vi "MC_7_12e_JW.vi"() -> ()   [LabVIEW 2011]
uses:
  <vilib>/Utility/file.llb/Read From Spreadsheet File (string).vi
  <vilib>/Utility/inputDevices.llb/keyboardAcquire.vi
  <vilib>/Utility/file.llb/Write To Spreadsheet File (DBL).vi
  <vilib>/Utility/file.llb/Write To Spreadsheet File (string).vi
  <vilib>/regexp/Match Regular Expression.xnode
panel:
  out "Rec: Temp":dbl
  out "Comments":string
  out "Folder Index":dbl caption="Length"
  out "Current \nRecord":string[](array[string])
  out "Transformer \nHeaders":string[](array[string])
  out "Current Device ID":string
  out "Column":string
  out "Row":string
  out "Rec: Concentration":dbl
  out "Rec: Solvent":string
  out "Rec: Method":string
  in  "?":T1(tab)
  out "Rec: Material":string
  in  "Treatment Concentration (mM):":dbl=30.0
  in  "Surface Treatment:":string
  in  "# Drops*:":dbl=inf
  in  "Solution Temp (C):":dbl=55.0
  in  "Relative Humidity (%):":dbl=nan
  in  "Room Temp (F):":dbl=nan
  in  "Time (s):":dbl=80.0
  out "Accel (RPM/s):":dbl
  in  "RPM:":dbl=1000.0
  in  "Wait Time (s):":dbl=10.0
  in  "Sample #:":dbl=1.0
  in  "Fabricator:":string="Jeremy"
  in  "Data File":path
  out "Data Folder":path
  in  "Image Folder":path
  out "Image File":path=path "D:/UserData/Desktop/Jeremy/WFU/Research/Programs/VI mods/Image Not Found.png"
  in  "Ramp (s):":dbl=3.0
  out "Calc: Trap Density-STS":dbl format="%#_4e"
  out "New: Trap Density-STS":dbl format="%#_4e"
  out "Rec: Trap Density-STS":dbl caption="Trap Density-STS" format="%#_3e"
  out "Calc: Trap Density-VT":dbl format="%#_4e"
  out "New: Trap Density-VT":dbl format="%#_4e"
  out "Rec: Trap Density-VT":dbl caption="Trap Density-VT" format="%#_3e"
  out "Calc: Onset V":dbl
  out "New: Onset":dbl
  out "Rec: Onset V":dbl caption="Onset V" format="%#_3g"
  out "Calc: Mobility-Lin":dbl format="%#_4e"
  out "New: Mobility-Lin":dbl format="%#_4e"
  out "Rec: Mobility-Lin":dbl caption="Mobility-Lin" format="%#_3e"
  out "Calc: Mobility-Sat":dbl format="%#_4e"
  out "Rec: Length":dbl caption="Length" format="%#_3g"
  out "Rec: Width":dbl caption="Width" format="%#_4g"
  out "Rec: Dielectric (d)":dbl caption="Dielectric (d)" format="%#_3g"
  out "XY Graph":cluster{dbl[], dbl[]}[](graph)
  in  "NumPts":dbl=5.0
  in  "Cancel Button":bool
  in  "Next Button":bool
  in  "Previous Button":bool
  in  "Up Button":bool
  in  "Down Button":bool
  out "Data Name:":string
  in  "Save Changes?":bool
  in  "New: Dielectric":dbl
  in  "New: Length":dbl
  in  "New: Width":dbl
  out "New: Mobility-Sat":dbl format="%#_4e"
  in  "Slide":dbl(slide) step=1.0 scale=-14.3..90.0 scale format="%#_1p"
  in  "Blank Button":bool
  in  "Zoom":i16(slide)=-3 scale=-5.0..5.0
  out "Image Out 2":T2(plugin-control)
  out "Image Out":T2(plugin-control)
  in  "Magnification":u16(ring) items=["5x", "10x", "20x", "50x", "80x"]
  out "Total Width":dbl
  out "Distances":dbl[](array[numeric])
  in  "Undo Button":bool
  in  "Remove Button":bool
  out "Rec: Mobility-Sat":dbl caption="Mobility-Sat" format="%#_3e"
  out "Index":string
  out "Image Name":string
  in  "Export":bool
  out "Calc: VT":dbl
  out "New: VT":dbl
  in  "Manual":bool
  out "XY Graph 2":cluster{dbl[], dbl[]}[](graph)
  in  "Next Button 2":bool
  in  "Previous Button 2":bool
  in  "Slide 2":dbl(slide) step=1.0 scale=-1.0..82.0 scale format="%#_1p"
  out "Calc: STS":dbl
  out "New: STS":dbl
  in  "NumPts 2":dbl=5.0 caption="NumPts"
  out "Rec: VT":dbl caption="Threshold V" format="%#_3g"
  out "Rec: STS":dbl caption="STS" format="%#_3g"
  out "Rec: On/Off":dbl caption="On/Off" format="%#_3e"
  in  "Save Changes? 2":bool
  in  "Save Changes? 3":bool
  out "Date Recorded":string="Date Recorded" caption="Recorded"
  out "Date Created":string caption="Fabricated"
  out "String":string
  in  "No Image":path=path "D:/UserData/Desktop/Jeremy/WFU/Research/Programs/VI mods/Image Not Found.png"
  in  "Project":path=path "D:/UserData/Desktop/Jeremy/WFU/Research/Programs/Mega Awesome/DeviceData.opj"
  out "Index 2":dbl
  out "Array 8":dbl[](array[numeric])
  out "Array 7":dbl[](array[numeric])
  out "ROI Descriptor out":T3 {"Contours"."Type" items=["No Selection", "Point", "Line", "Rectangle", "Oval", "Polygon", "Freehand Region", "Annulus", "Unused2", "Unused3", "Broken Line", "Freehand Line", "Rotated Rectangle"]}
  out "ROI Descriptor":T3 {"Contours"."Type" items=["No Selection", "Point", "Line", "Rectangle", "Oval", "Polygon", "Freehand Region", "Annulus", "Unused2", "Unused3", "Broken Line", "Freehand Line", "Rotated Rectangle"]}
  out "Numeric 3":dbl
  out "Array 6":dbl[][](array[numeric])
  out "Cluster":T4
  out "Array 5":dbl[](array[numeric])
  out "Array 4":dbl[](array[numeric])
  out "Array 3":dbl[](array[numeric])
  out "Numeric 2":dbl
  out "Numeric":dbl
  out "Array 2":dbl[](array[numeric])
  out "Array":dbl[](array[numeric])
  out "MobVi Index":dbl
  out "Table Control 2":string[][](table)
  out "Table Control":string[][](table)
  in  "Row Start":dbl=20.0
  # "Data Locations"
  # "Data Location"
  # "Image Location"
  # "Sample Properties"
  # "*     Inf = Full coverage\n   NaN = Unknown or Not Applicable"
  # "Recorded"
  # "Calculated"
  # "Re-Calculated"
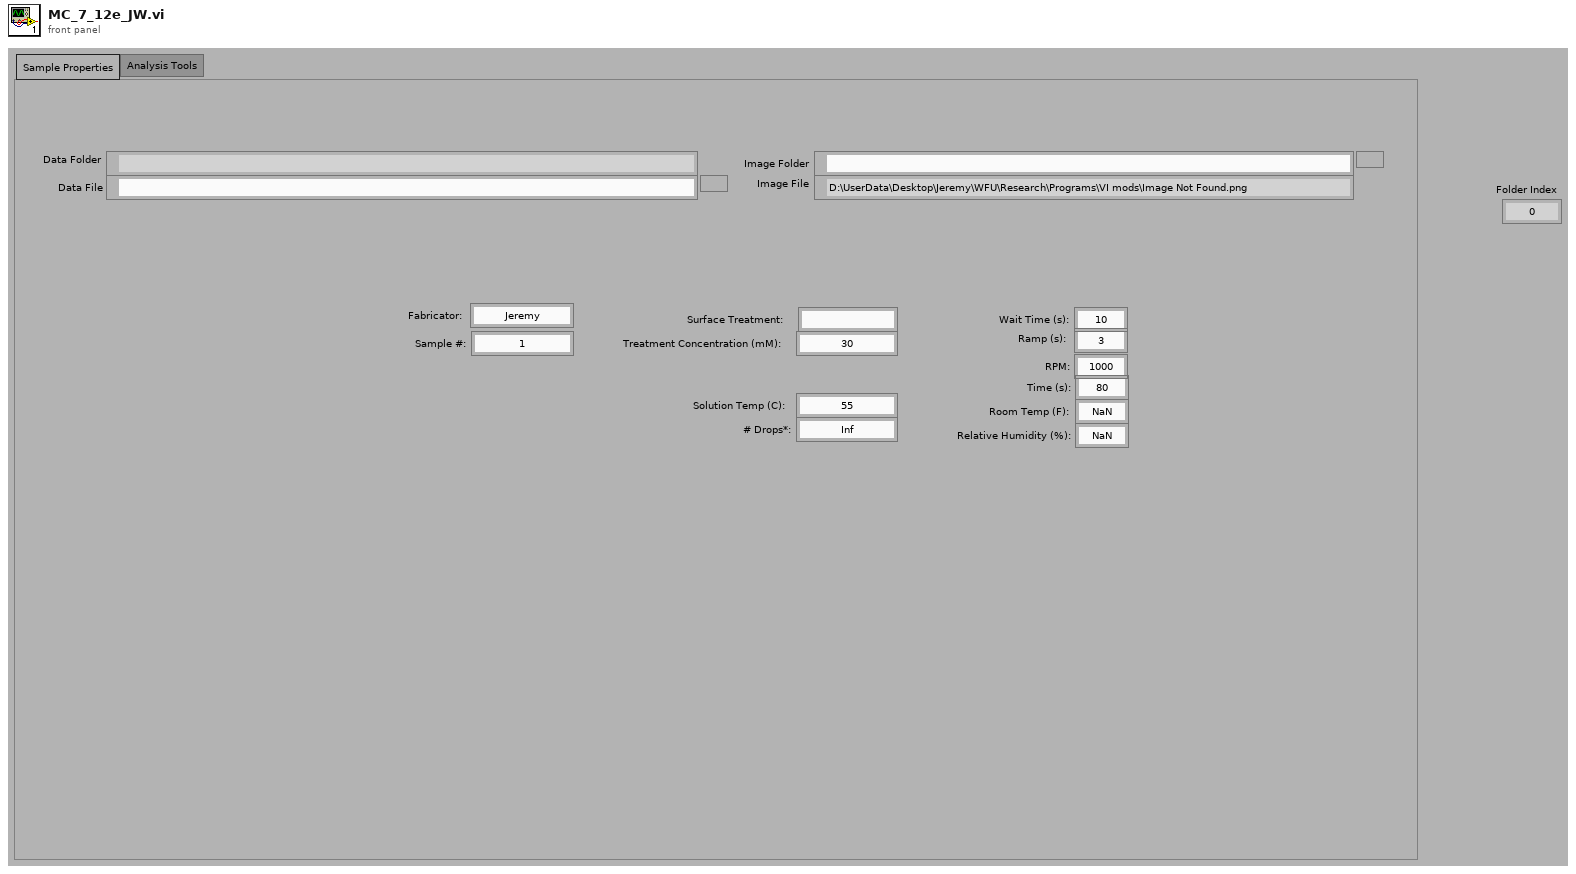
[diagram p1: front panel]
types:
  T1 = enum32{"Sample Properties", "Analysis Tools", "Current Database"}
  T2 = typedef "IMAQ Image.ctl" = refnum<image>
  T3 = typedef "ROI Descriptor" = cluster{"Global Rectangle":i32[], "Contours":cluster{"ID":enum32{"External", "Internal"}, "Type":u32, "Coordinates":i32[]}[]}
  T4 = cluster{"Numeric":dbl, "Numeric 2":dbl, "Numeric 3":dbl, "Numeric 4":dbl}
  T5 = cluster{"Mobility-Sat":dbl, "Moblitity-Lin":dbl, "On/Off":dbl, "Threshold Voltage":dbl, "Onset Voltage":dbl, "STS":dbl, "Trap Density-VT":dbl, "Trap Density-STS":dbl}
  T6 = cluster{"Date Recorded":string, "Index":string, "Length":dbl, "Width":dbl, "Sample Temp":dbl}
  T7 = cluster{"Date Created":string, "Material":string, "Solvent":string, "Concentration":dbl, "Method":string, "Dielectric (nm)":dbl, "Treatment":string, "Comments":string}
  T8 = cluster{"[0]":cluster{dbl[], dbl[]}, "[1]":cluster{dbl[], dbl[]}, "[2]":cluster{dbl[], dbl[]}, "[3]":cluster{dbl[], dbl[]}, "[4]":cluster{dbl[], dbl[]}, "[5]":cluster{dbl[], dbl[]}, "[6]":cluster{dbl[], dbl[]}, "[7]":cluster{dbl[], dbl[]}, "[8]":cluster{dbl[], dbl[]}}
  T9 = cluster{"Global Rectangle":i32[], "Contours":cluster{"Contour Type":u32, "ROI Type":u32, "Points":i32[]}[]}
  T10 = typedef "LVBoundsTypeDef.ctl" = cluster{"Width":u32, "Height":u32}
  T11 = enum16{"0", "1", "2", "3", "4", "5", "6", "7", "8", "9", "A", "B", "C", "D", "E", "F", "G", "H", "I", "J", "K", "L", "M", "N", "O", "P", "Q", "R", "S", "T", "U", "V", "W", "X", "Y", "Z", "F1", "F2", "F3", "F4", "F5", "F6", "F7", "F8", "F9", "F10", "F11", "F12", "F13", "F14", "F15", "ADD", "BACK", "BACKSLASH", "CAPITAL", "COMMA", "DECIMAL", "DELETE", "DIVIDE", "DOWN", "END", "EQUALS", "ESCAPE", "GRAVE (`)", "HOME", "INSERT", "LBRACKET", "LCONTROL", "LEFT", "L ALT", "LSHIFT", "LWIN", "MINUS", "MULTIPLY", "NEXT", "NUMLOCK", "NUMPAD_0", "NUMPAD_1", "NUMPAD_2", "NUMPAD_3", "NUMPAD_4", "NUMPAD_5", "NUMPAD_6", "NUMPAD_7", "NUMPAD_8", "NUMPAD_9", "PAUSE", "PERIOD", "PRIOR (PG UP)", "RBRACKET", "RCONTROL", "RETURN", "RIGHT", "R ALT", "RSHIFT", "RWIN", "SCROLL", "SEMICOLON", "SLASH", "SPACE", "SUBTRACT", "TAB", "UP", "ENTER (num pad)", "' (quote)"}[]
  T12 = cluster{"Contour Type":u32, "ROI Type":u32, "Points":i32[]}[]
  T13 = cluster{i32[], cluster{"Contour Type":u32, "ROI Type":u32, "Points":i32[]}[]}
  T14 = enum16{"0", "1", "2", "3", "4", "5", "6", "7", "8", "9", "A", "B", "C", "D", "E", "F", "G", "H", "I", "J", "K", "L", "M", "N", "O", "P", "Q", "R", "S", "T", "U", "V", "W", "X", "Y", "Z", "F1", "F2", "F3", "F4", "F5", "F6", "F7", "F8", "F9", "F10", "F11", "F12", "F13", "F14", "F15", "ADD", "BACK", "BACKSLASH", "CAPITAL", "COMMA", "DECIMAL", "DELETE", "DIVIDE", "DOWN", "END", "EQUALS", "ESCAPE", "GRAVE (`)", "HOME", "INSERT", "LBRACKET", "LCONTROL", "LEFT", "L ALT", "LSHIFT", "LWIN", "MINUS", "MULTIPLY", "NEXT", "NUMLOCK", "NUMPAD_0", "NUMPAD_1", "NUMPAD_2", "NUMPAD_3", "NUMPAD_4", "NUMPAD_5", "NUMPAD_6", "NUMPAD_7", "NUMPAD_8", "NUMPAD_9", "PAUSE", "PERIOD", "PRIOR (PG UP)", "RBRACKET", "RCONTROL", "RETURN", "RIGHT", "R ALT", "RSHIFT", "RWIN", "SCROLL", "SEMICOLON", "SLASH", "SPACE", "SUBTRACT", "TAB", "UP", "ENTER (num pad)", "' (quote)"}
  T15 = cluster{string, sgl, bool, bool, bool, bool, bool, bool, i32}
  T16 = cluster{i32, cluster{string, sgl, bool, bool, bool, bool, bool, bool, i32}, i32, i32}
  T17 = cluster{"Contour Type":u32, "ROI Type":u32, "Points":i32[]}
  T18 = cluster{"Points[0]":i32, "Points[1]":i32, "Points[2]":i32, "Points[3]":i32, "Points[4]":i32, "Points[5]":i32, "Points[6]":i32, "Points[7]":i32, "Points[8]":i32}
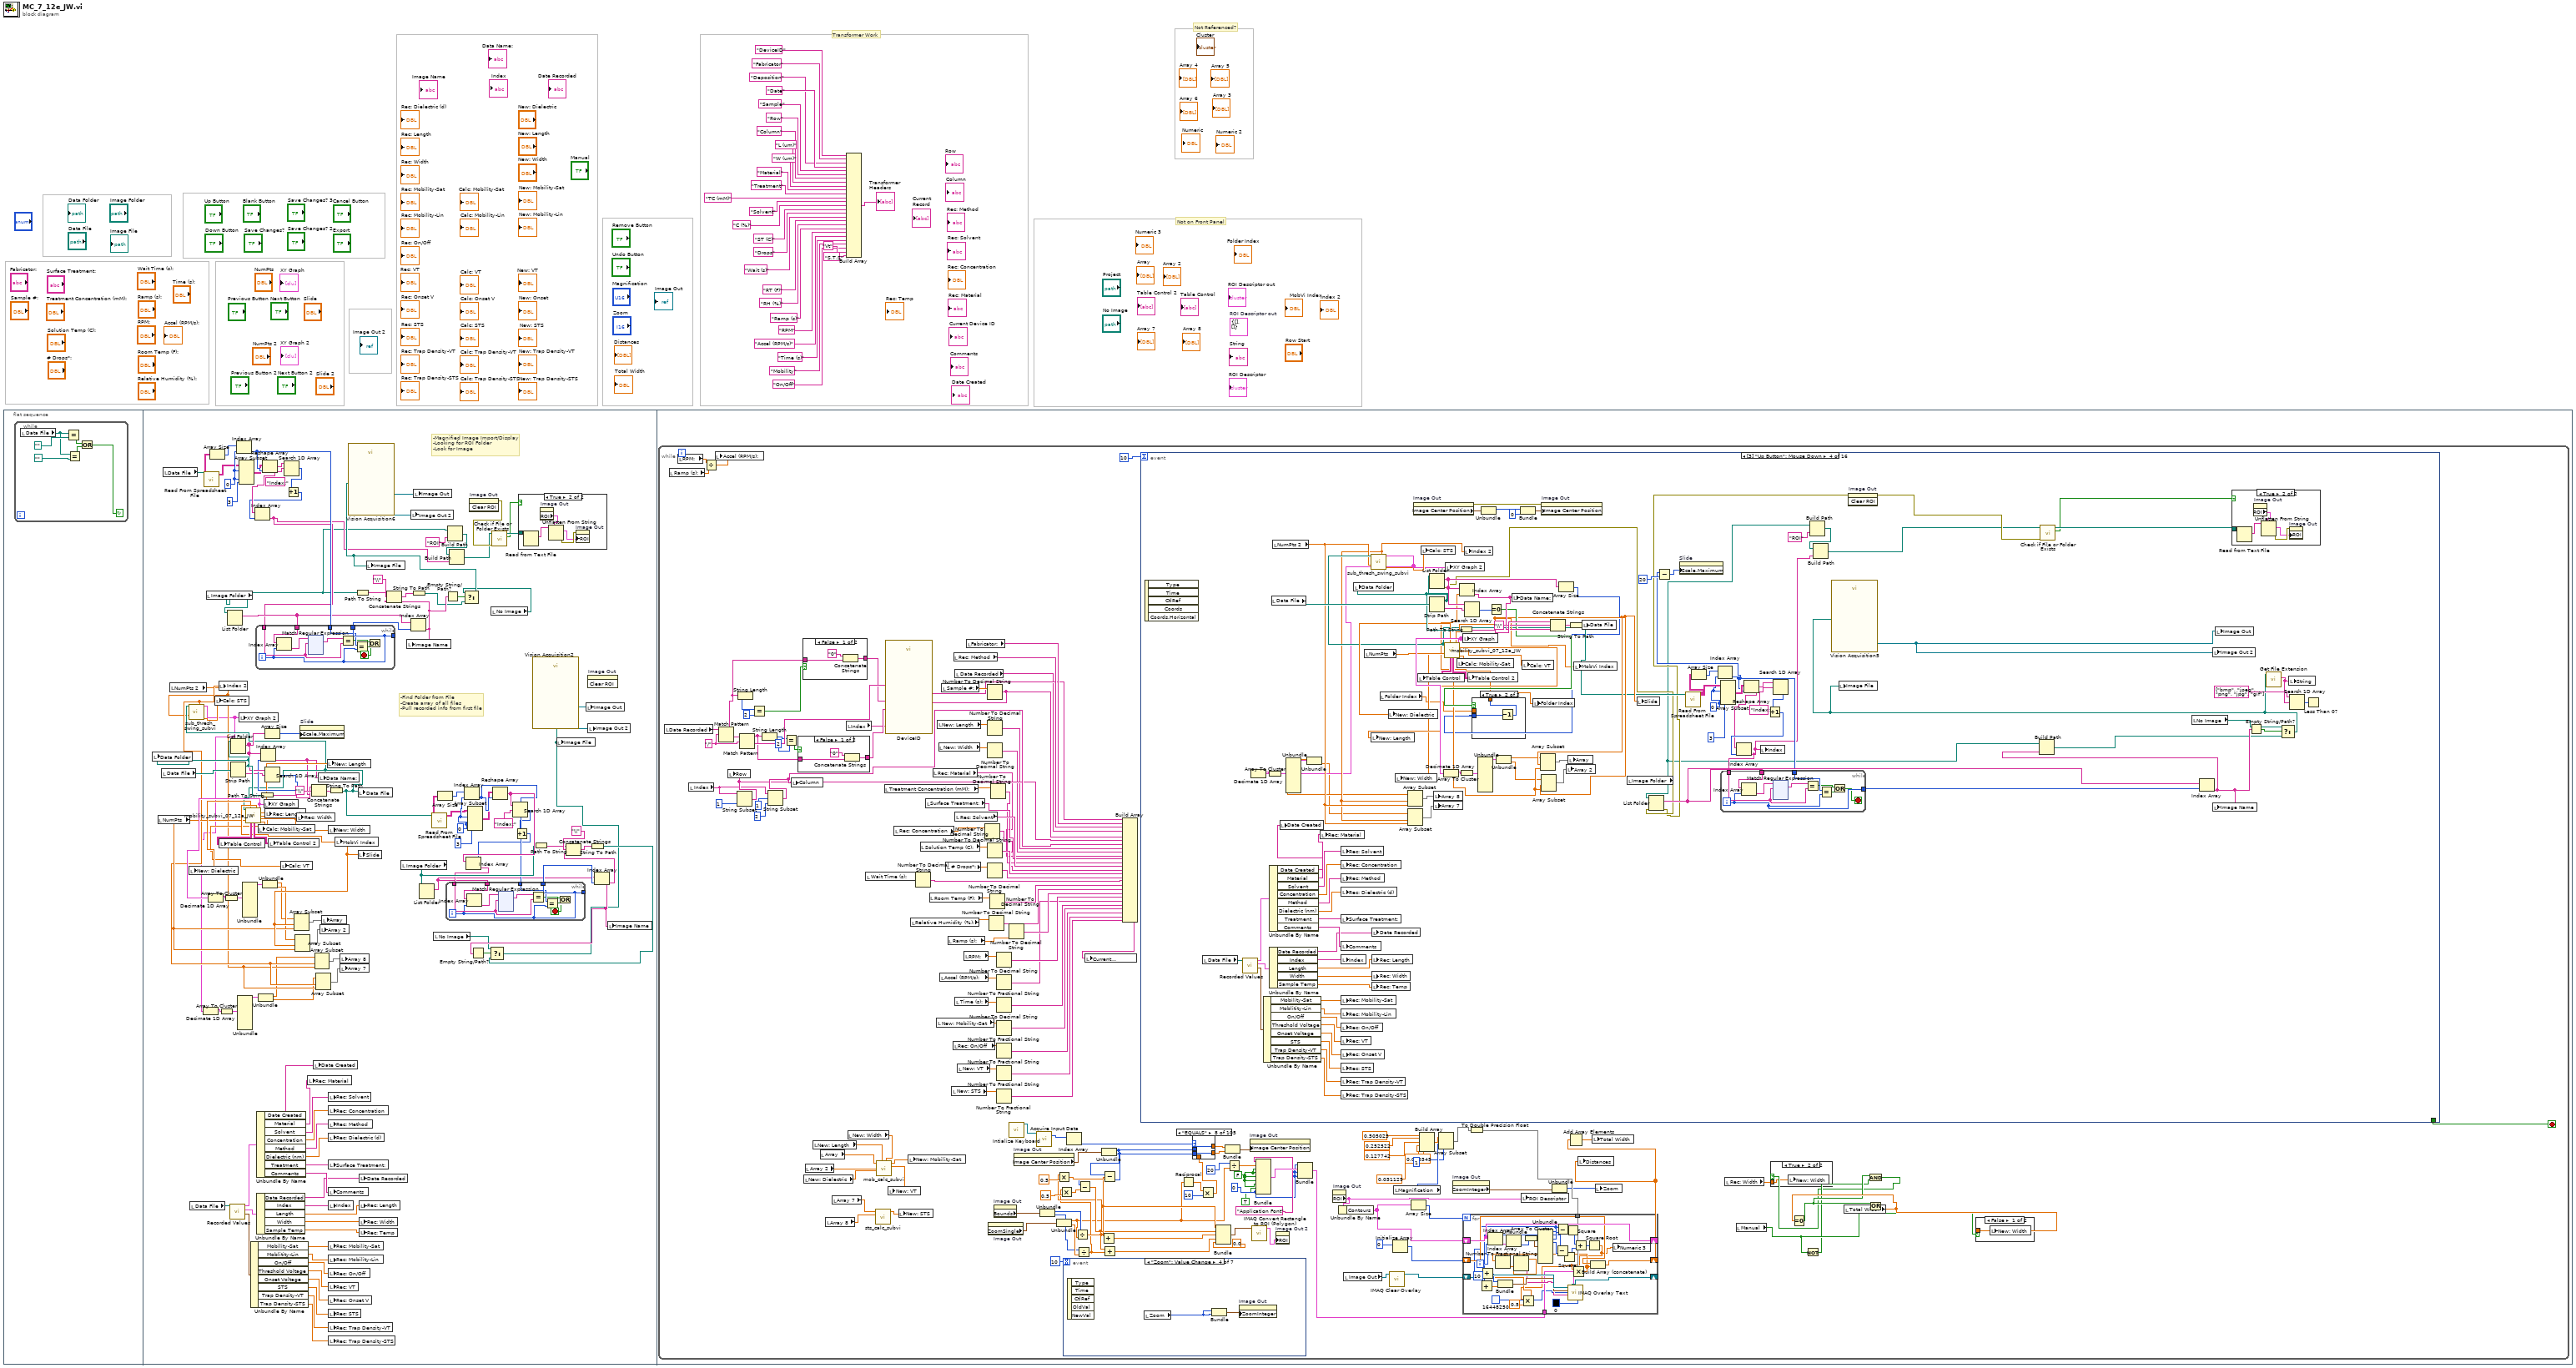
[diagram p0: block diagram]
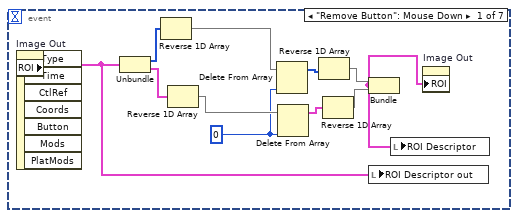
[diagram p7: hidden frame]
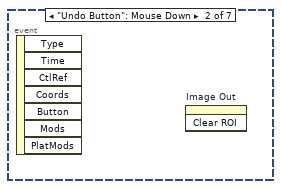
[diagram p8: hidden frame]
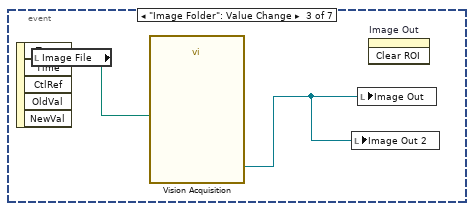
[diagram p9: hidden frame]
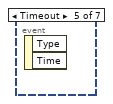
[diagram p10: hidden frame]
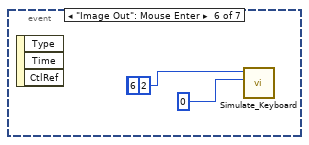
[diagram p11: hidden frame]
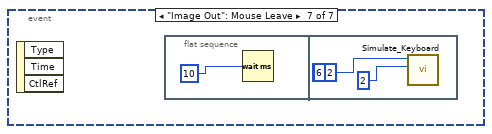
[diagram p12: hidden frame]
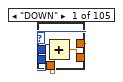
[diagram p13: hidden frame]
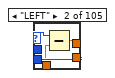
[diagram p14: hidden frame]
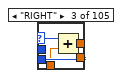
[diagram p15: hidden frame]
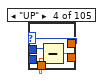
[diagram p16: hidden frame]
diagram:
  (unwired) T3 {"Global Rectangle"=[], "Contours"=[]}  # ROI Descriptor out
  # "Not Referenced?"
  # "Transformer Work"
  # "Not on Front Panel"
  n1 = flat-sequence {
    frame #0 {
      n2 = while {
        stop <- w29 continue-if-true
        n3 = local read "Data File"() -> (w31:path)
        n4 = Equal?(x=w31, y=path "") -> (x = y?=w33:bool)
        n5 = Equal?(x=w31, y=path "") -> (x = y?=w32:bool)
        n6 = Or(x=w33, y=w32) -> (x .or. y?=w29:bool)
      }
    }
    frame #1 {
      w115 = 0
      w140 = 0
      # "-Find Folder from File\n-Create array of all files\n-Pull recorded info from first file"
      # "-Magnified Image Import/Display\n-Looking for ROI Folder\n-Look for Image"
      n7 = local read "NumPts"() -> (w91:dbl)
      n8 = local read "Data File"() -> (w119:path)
      n9 = local read "Data File"() -> (w135:path)
      n10 = local read "NumPts 2"() -> (w86:dbl)
      n11 = local read "Data File"() -> (w59:path)
      n12 = call-poly <vilib>:"Read From Spreadsheet File.vi"("file path (dialog if empty)"=w135) -> ("all rows"=w138:string[][])  [unwired: 6 in, 4 out]
      n13 = local read "Image Folder"() -> (w61:path)
      n14 = Array Size(array=w138) -> (size(s)=w139:i32[])
      n15 = List Folder(path=w61) -> (filenames=w144:string[])  [unwired: 3 in, 3 out]
      n16 = call "Recorded Values.vi"("Path"=w59) -> ("Recorded Char"=w57:T5, "Recorded Prop"=w56:T6, "Fabrication Prop"=w58:T7)  [unwired: 8 in]
      n17 = Strip Path(path=w119) -> (stripped path=w120:path, name=w102:string)
      n18 = local write "Data Folder"(w120) -> ()
      n19 = List Folder(path=w120) -> (filenames=w109:string[])  [unwired: 3 in, 3 out]
      n20 = Index Array(array=w139, index=w140) -> (element=w146:i32)
      n21 = Array Subset(array=w138, index (row)=w140, index (col)=w140, length (col)=3) -> (w137:string[][])  [unwired: 1 in]
      n22 = Unbundle By Name(w57) -> ("Mobility-Sat"=w43:dbl, "Moblitity-Lin"=w42:dbl, "On/Off"=w41:dbl, "Threshold Voltage"=w40:dbl, "Onset Voltage"=w39:dbl, "STS"=w38:dbl, "Trap Density-VT"=w37:dbl, "Trap Density-STS"=w36:dbl)
      n23 = Unbundle By Name(w58) -> ("Date Created"=w35:string, "Material"=w55:string, "Solvent"=w54:string, "Concentration"=w53:dbl, "Method"=w52:string, "Dielectric (nm)"=w51:dbl, "Treatment"=w50:string, "Comments"=w49:string)
      n24 = Unbundle By Name(w56) -> ("Date Recorded"=w48:string, "Index"=w47:string, "Length"=w46:dbl, "Width"=w45:dbl, "Sample Temp"=w44:dbl)
      n25 = Path To String(path=w120) -> (string=w101:string)
      n26 = Reshape Array(w137, w146) -> (w151:string[])
      n27 = Array Size(array=w109) -> (size(s)=w110:i32)
      n28 = Search 1D Array(1D array=w109, element=w102) -> (index of element=w108:i32)  [unwired: 1 in]
      n29 = Index Array(array=w109, index=w108) -> (element=w60:string)
      n30 = Search 1D Array(1D array=w151, element="Index:") -> (index of element=w143:i32)  [unwired: 1 in]
      n31 = Increment(x=w143) -> (x+1=w142:i32)
      n32 = Index Array(array=w151, index=w142) -> (element=w62:string)
      n33 = while {
        tunnel: w144 -> [w284]
        tunnel: w62 -> [w282]
        tunnel: [w281] -> _
        tunnel: [w281] -> w145
        tunnel: w146 -> [w280]
        i -> [w281]
        stop <- w277 stop-if-true
        n34 = Index Array(array=w284, index=w281) -> (element=w285:string)
        n35 = xnode "Match Regular Expression"("input string"=w285, "regular expression"=w282) -> ("whole match"=w283:string)  [unwired: 4 in, 4 out]
        n36 = Equal?(x=w283, y=w282) -> (x = y?=w279:bool)
        n37 = Equal?(x=w280, y=w281) -> (x = y?=w278:bool)
        n38 = Or(x=w279, y=w278) -> (x .or. y?=w277:bool)
      }
      n39 = property on="Slide" class="Slide (strict)"("Scale.Maximum"=w110) -> ()  [unwired: 2 in, 2 out]
      n40 = local write "Rec: Material"(w55) -> ()
      n41 = Concatenate Strings(w101, "\\", w60) -> (w103:string)
      n42 = local write "Date Created"(w35) -> ()
      n43 = local write "Data Name:"(w60) -> ()
      n44 = local write "Rec: Solvent"(w54) -> ()
      n45 = local write "Rec: Concentration"(w53) -> ()
      n46 = local write "Rec: Method"(w52) -> ()
      n47 = local write "Rec: Dielectric (d)"(w51) -> ()
      n48 = local write "Surface Treatment:"(w50) -> ()
      n49 = local write "Comments"(w49) -> ()
      n50 = local write "Index"(w47) -> ()
      n51 = local write "Rec: Mobility-Sat"(w43) -> ()
      n52 = local write "Rec: Mobility-Lin"(w42) -> ()
      n53 = local write "Rec: On/Off"(w41) -> ()
      n54 = local write "Rec: VT"(w40) -> ()
      n55 = local write "Rec: Onset V"(w39) -> ()
      n56 = local write "Rec: STS"(w38) -> ()
      n57 = local write "Rec: Trap Density-VT"(w37) -> ()
      n58 = local write "Rec: Trap Density-STS"(w36) -> ()
      n59 = String To Path(string=w103) -> (path=w92:path)
      n60 = call "sub_thresh_swing_subvi.vi"("Path"=w92, "NumPts"=w86) -> ("Index"=w87:dbl, "XY Graph"=w82:cluster{dbl[], dbl[]}[], "Sub Threshold Swing"=w93:dbl)  [unwired: 9 in, 2 out]
      n61 = Decimate 1D Array(w82) -> (w83:cluster{dbl[], dbl[]}[])  [unwired: 1 out]
      n62 = local write "Calc: STS"(w93) -> ()
      n63 = local write "Index 2"(w87) -> ()
      n64 = Array To Cluster(array=w83) -> (cluster=w85:T8)
      n65 = Unbundle(w85) -> ("[0]"=w84:cluster{dbl[], dbl[]})  [unwired: 8 out]
      n66 = local write "XY Graph 2"(w82) -> ()
      n67 = call "mobility_subvi_07_12a_JW.vi"("Path"=w92, "NumPts"=w91) -> ("Dielectric (d)"=w97:dbl, "Index"=w98:dbl, "XY Graph"=w134:cluster{dbl[], dbl[]}[], "Length"=w96:dbl, "Vt"=w94:dbl, "Width"=w95:dbl, "Table Control"=w105:string[][], "Table Control 2"=w106:string[][], "Mobility"=w107:dbl)  [unwired: 4 in, 1 out]
      n68 = local write "New: Dielectric"(w97) -> ()
      n69 = Decimate 1D Array(w134) -> (w133:cluster{dbl[], dbl[]}[])  [unwired: 1 out]
      n70 = local write "Table Control"(w105) -> ()
      n71 = Array To Cluster(array=w133) -> (cluster=w131:T8)
      n72 = Unbundle(w131) -> ("[0]"=w132:cluster{dbl[], dbl[]})  [unwired: 8 out]
      n73 = local write "Calc: Mobility-Sat"(w107) -> ()
      n74 = Unbundle(w84) -> (w80:dbl[], w79:dbl[])
      n75 = Unbundle(w132) -> (w81:dbl[], w88:dbl[])
      n76 = local write "XY Graph"(w134) -> ()
      n77 = local write "Rec: Length"(w96) -> ()
      n78 = local write "Table Control 2"(w106) -> ()
      n79 = local write "Calc: VT"(w94) -> ()
      n80 = Array Subset(array=w81, index=w98, length=w91) -> (w99:dbl[])
      n81 = Array Subset(array=w88, index=w98, length=w91) -> (w100:dbl[])
      n82 = local write "Rec: Width"(w95) -> ()
      n83 = Array Subset(array=w80, index=w87, length=w86) -> (w90:dbl[])
      n84 = Array Subset(array=w79, index=w87, length=w86) -> (w89:dbl[])
      n85 = local write "Array 2"(w100) -> ()
      n86 = local write "Array"(w99) -> ()
      n87 = local write "New: Length"(w96) -> ()
      n88 = local write "New: Width"(w95) -> ()
      n89 = local write "MobVi Index"(w98) -> ()
      n90 = local write "Array 8"(w90) -> ()
      n91 = local write "Array 7"(w89) -> ()
      n92 = Path To String(path=w61) -> (string=w148:string)
      n93 = local write "Data File"(w92) -> ()
      n94 = local write "Slide"(w98) -> ()
      n95 = local write "Date Recorded"(w48) -> ()
      n96 = local write "Rec: Length"(w46) -> ()
      n97 = local write "Rec: Width"(w45) -> ()
      n98 = local write "Rec: Temp"(w44) -> ()
      n99 = local read "Image Folder"() -> (w126:path)
      n100 = Index Array(array=w144, index=w145) -> (element=w78:string)
      n101 = Concatenate Strings(w148, "\\", w78) -> (w149:string)
      n102 = local write "Image Name"(w78) -> ()
      n103 = String To Path(string=w149) -> (path=w76:path)
      n104 = List Folder(path=w126) -> (filenames=w122:string[])  [unwired: 3 in, 3 out]
      n105 = call-poly <vilib>:"Read From Spreadsheet File.vi"("file path (dialog if empty)"=w92) -> ("all rows"=w113:string[][])  [unwired: 6 in, 4 out]
      n106 = local read "No Image"() -> (w70:path)
      n107 = Array Size(array=w113) -> (size(s)=w114:i32[])
      n108 = Empty String/Path?(string/path=w78) -> (empty?=w77:bool)
      n109 = Build Path(base path=w61, name or relative path="ROI") -> (appended path=w64:path)
      n110 = Build Path(base path=w64, name or relative path=w62) -> (appended path=w63:path)
      n111 = Index Array(array=w114, index=w115) -> (element=w125:i32)
      n112 = Array Subset(array=w113, index (row)=w115, index (col)=w115, length (col)=3) -> (w112:string[][])  [unwired: 1 in]
      n113 = invoke on="Image Out" class="ImageControl" method="Clear ROI"() -> (error out=w68:errorcluster)  [unwired: 3 in, 2 out]
      n114 = local read "No Image"() -> (w69:path)
      n115 = Select(t=w69, s=w77, f=w76) -> (s? t:f=w75:path)
      n116 = call "Vision Acquisition6"("Image Path"=w75) -> ("Image Out"=w147:T2)  [unwired: 25 in, 1 out]
      n117 = local write "Image File"(w75) -> ()
      n118 = local write "Image Out 2"(w147) -> ()
      n119 = local write "Image Out"(w147) -> ()
      n120 = call <vilib>:"Check if File or Folder Exists.vi"("error in (no error)"=w68, "path"=w63) -> ("file or folder exists?"=w66:bool, "dup path"=w67:path)  [unwired: 7 in, 1 out]
      n121 = Reshape Array(w112, w125) -> (w130:string[])
      n122 = Search 1D Array(1D array=w130, element="Index:") -> (index of element=w118:i32)  [unwired: 1 in]
      n123 = Increment(x=w118) -> (x+1=w117:i32)
      n124 = Index Array(array=w130, index=w117) -> (element=w123:string)
      n125 = while {
        tunnel: w122 -> [w164]
        tunnel: w123 -> [w162]
        tunnel: [w161] -> _
        tunnel: [w161] -> w124
        tunnel: w125 -> [w160]
        i -> [w161]
        stop <- w157 stop-if-true
        n126 = Index Array(array=w164, index=w161) -> (element=w165:string)
        n127 = xnode "Match Regular Expression"("input string"=w165, "regular expression"=w162) -> ("whole match"=w163:string)  [unwired: 4 in, 4 out]
        n128 = Equal?(x=w163, y=w162) -> (x = y?=w159:bool)
        n129 = Equal?(x=w160, y=w161) -> (x = y?=w158:bool)
        n130 = Or(x=w159, y=w158) -> (x .or. y?=w157:bool)
      }
      n131 = case shown="True" w66 {
        tunnel: w67 -> [_ w152]
        frame False {
        }
        frame True {
          n132 = Read from Text File(file (use dialog)=w152) -> (text=w156:string)  [unwired: 3 in, 3 out]
          n133 = property on="Image Out" class="ImageControl"() -> ("ROI"=w153:T9)  [unwired: 2 in, 2 out]
          n134 = Unflatten From String(type=w153, binary string=w156) -> (value=w154:T9, error out=w155:errorcluster)  [unwired: 3 in, 1 out]
          n135 = property on="Image Out" class="ImageControl"(error in=w155, "ROI"=w154) -> ()  [unwired: 1 in, 2 out]
        }
      }
      n136 = Path To String(path=w126) -> (string=w127:string)
      n137 = invoke on="Image Out" class="ImageControl" method="Clear ROI"() -> ()  [unwired: 3 in, 3 out]
      n138 = Index Array(array=w122, index=w124) -> (element=w73:string)
      n139 = Empty String/Path?(string/path=w73) -> (empty?=w74:bool)
      n140 = Concatenate Strings(w127, "\\", w73) -> (w128:string)
      n141 = String To Path(string=w128) -> (path=w72:path)
      n142 = Select(t=w70, s=w74, f=w72) -> (s? t:f=w71:path)
      n143 = call "Vision Acquisition2"("Image Path"=w71) -> ("Image Out"=w121:T2)  [unwired: 25 in, 1 out]
      n144 = local write "Image File"(w71) -> ()
      n145 = local write "Image Out"(w121) -> ()
      n146 = local write "Image Out 2"(w121) -> ()
      n147 = local write "Image Name"(w73) -> ()
    }
    frame #2 {
      n148 = while {
        stop <- w544 stop-if-true
        w430 = "/"
        w494 = FALSE
        w492 = 0
        n149 = local read "Date Recorded"() -> (w433:string)
        n150 = local read "Ramp (s):"() -> (w400:dbl)
        n151 = local read "RPM:"() -> (w401:dbl)
        n152 = local read "Index"() -> (w403:string)
        n153 = Divide(x=w401, y=w400) -> (x/y=w399:dbl)
        n154 = local write "Accel (RPM/s):"(w399) -> ()
        n155 = Match Pattern(string=w433, regular expression=w430) -> (before substring=w424:string, after substring=w431:string)  [unwired: 1 in, 2 out]
        n156 = String Subset(string=w403, length (rest)=1) -> (substring=w458:string)  [unwired: 1 in]
        n157 = local write "Row"(w458) -> ()
        n158 = String Length(string=w424) -> (length=w427:i32)
        n159 = Match Pattern(string=w431, regular expression=w430) -> (before substring=w418:string, after substring=w429:string)  [unwired: 1 in, 2 out]
        n160 = Equal?(x=w427, y=2) -> (x = y?=w425:bool)
        n161 = String Length(string=w418) -> (length=w420:i32)
        n162 = String Subset(string=w403, offset (0)=1, length (rest)=2) -> (substring=w459:string)
        n163 = Equal?(x=w420, y=2) -> (x = y?=w422:bool)
        n164 = local write "Column"(w459) -> ()
        n165 = case shown="False" w422 {
          tunnel: w418 -> [w546 w548]
          tunnel: [w545 w548] -> w419
          frame False {
            n166 = Concatenate Strings("0", w546) -> (w545:string)
          }
          frame True {
          }
        }
        n167 = case shown="False" w425 {
          tunnel: w424 -> [w550 w552]
          tunnel: [w549 w552] -> w423
          frame False {
            n168 = Concatenate Strings("0", w550) -> (w549:string)
          }
          frame True {
          }
        }
        n169 = local read "New: Dielectric"() -> (w482:dbl)
        n170 = local read "Array 2"() -> (w478:dbl[])
        n171 = local read "New: Length"() -> (w480:dbl)
        n172 = local read "Array"() -> (w479:dbl[])
        n173 = local read "Array 8"() -> (w474:dbl[])
        n174 = local read "Array 7"() -> (w475:dbl[])
        n175 = local read "Index"() -> (w417:string)
        n176 = local read "New: Width"() -> (w483:dbl)
        n177 = local read "Wait Time (s):"() -> (w463:dbl)
        n178 = call "sts_calc_subvi.vi"("Array 2"=w474, "Array"=w475) -> ("STS"=w476:dbl)  [unwired: 9 in]
        n179 = call "mob_calc_subvi.vi"("Width"=w483, "Length"=w480, "Dielectric (d)"=w482, "Array 2"=w478, "Array"=w479) -> ("Vt"=w477:dbl, "Mobility"=w481:dbl)  [unwired: 4 in, 1 out]
        n180 = local read "Treatment Concentration (mM):"() -> (w411:dbl)
        n181 = local write "New: VT"(w477) -> ()
        n182 = local read "Rec: Concentration"() -> (w398:dbl)
        n183 = local write "New: STS"(w476) -> ()
        n184 = local write "New: Mobility-Sat"(w481) -> ()
        n185 = local read "Relative Humidity (%):"() -> (w408:dbl)
        n186 = Number To Decimal String(number=w463) -> (decimal integer string=w464:string)  [unwired: 1 in]
        n187 = local read "Solution Temp (C):"() -> (w452:dbl)
        n188 = local read "Surface Treatment:"() -> (w410:string)
        n189 = local read "Room Temp (F):"() -> (w456:dbl)
        n190 = local read "Rec: Material"() -> (w406:string)
        n191 = local read "New: Mobility-Sat"() -> (w445:dbl)
        n192 = local read "New: Length"() -> (w416:dbl)
        n193 = local read "New: Width"() -> (w415:dbl)
        n194 = local read "Accel (RPM/s):"() -> (w443:dbl)
        n195 = local read "Sample #:"() -> (w435:dbl)
        n196 = local read "# Drops*:"() -> (w453:dbl)
        n197 = local read "Ramp (s):"() -> (w461:dbl)
        n198 = local read "New: STS"() -> (w437:dbl)
        n199 = local read "Rec: On/Off"() -> (w441:dbl)
        n200 = local read "Rec: Method"() -> (w436:string)
        n201 = local read "Date Recorded"() -> (w432:string)
        n202 = local read "Rec: Solvent"() -> (w412:string)
        n203 = local read "Time (s):"() -> (w448:dbl)
        n204 = local read "New: VT"() -> (w439:dbl)
        n205 = local read "RPM:"() -> (w449:dbl)
        n206 = local read "Fabricator:"() -> (w457:string)
        n207 = Number To Decimal String(number=w398) -> (decimal integer string=w397:string)  [unwired: 1 in]
        n208 = Number To Decimal String(number=w453) -> (decimal integer string=w454:string)  [unwired: 1 in]
        n209 = Number To Decimal String(number=w435) -> (decimal integer string=w428:string)  [unwired: 1 in]
        n210 = call "DeviceID"("Sample"=w428, "Year"=w429, "Month"=w423, "Day"=w419, "Index"=w417) -> ("Result"=w434:string)  [unwired: 9 in, 1 out]
        n211 = Number To Decimal String(number=w416) -> (decimal integer string=w414:string)  [unwired: 1 in]
        n212 = Number To Decimal String(number=w415) -> (decimal integer string=w413:string)  [unwired: 1 in]
        n213 = Number To Decimal String(number=w452) -> (decimal integer string=w451:string)  [unwired: 1 in]
        n214 = property on="Image Out" class="ImageControl"() -> ("ZoomSingle"=w512:cluster{"X":sgl, "Y":sgl})  [unwired: 2 in, 2 out]
        n215 = Number To Decimal String(number=w408) -> (decimal integer string=w407:string)  [unwired: 1 in]
        n216 = Number To Decimal String(number=w456) -> (decimal integer string=w455:string)  [unwired: 1 in]
        n217 = Number To Decimal String(number=w411) -> (decimal integer string=w409:string)  [unwired: 1 in]
        n218 = property on="Image Out" class="ImageControl"() -> ("Bounds"=w513:T10)  [unwired: 2 in, 2 out]
        n219 = Number To Decimal String(number=w449) -> (decimal integer string=w450:string)  [unwired: 1 in]
        n220 = Number To Fractional String(number=w443) -> (F-format string=w444:string)  [unwired: 3 in]
        n221 = Number To Decimal String(number=w448) -> (decimal integer string=w447:string)  [unwired: 1 in]
        n222 = Number To Fractional String(number=w445) -> (F-format string=w446:string)  [unwired: 3 in]
        n223 = Number To Fractional String(number=w441) -> (F-format string=w442:string)  [unwired: 3 in]
        n224 = Number To Fractional String(number=w439) -> (F-format string=w440:string)  [unwired: 3 in]
        n225 = Number To Fractional String(number=w437) -> (F-format string=w438:string)  [unwired: 3 in]
        n226 = Number To Decimal String(number=w461) -> (decimal integer string=w462:string)  [unwired: 1 in]
        n227 = call <vilib>:"Intialize Keyboard.vi"() -> ("device ID"=w524:refnum<k1>)  [unwired: 10 in, 1 out]
        n228 = property on="Image Out" class="ImageControl"() -> ("Image Center Position"=w519:cluster{"X":u32, "Y":u32})  [unwired: 2 in, 2 out]
        n229 = call-poly <vilib>:"Acquire Input Data.vi"("device ID"=w524) -> ("keys pressed"=w523:T11)  [unwired: 16 in, 2 out]
        n230 = Unbundle(w513) -> ("Width"=w510:u32, "Height"=w509:u32)
        n231 = Unbundle(w512) -> ("X"=w487:sgl, "Y"=w511:sgl)
        n232 = event shown="[3] \"Zoom\": Value Change" {
          selector: _ -> [_ _ _ _ _ _ _]
          dyn-events: _ -> [_ _ _ _ _ _ _]
          timeout: 10 -> [_ _ _ _ _ _ _]
          event "Remove Button": Mouse Down {
            w557 = 0
            n233 = property on="Image Out" class="ImageControl"() -> ("ROI"=w555:T9)  [unwired: 2 in, 2 out]
            n234 = event-data() -> ()  [unwired: 1 in, 7 out]
            n235 = Unbundle(w555) -> ("Global Rectangle"=w558:i32[], "Contours"=w560:T12)
            n236 = Reverse 1D Array(array=w558) -> (reversed array=w559:i32[])
            n237 = Reverse 1D Array(array=w560) -> (reversed array=w561:T12)
            n238 = Delete From Array(array=w559, index=w557) -> (array with subset deleted=w562:i32[])  [unwired: 1 in, 1 out]
            n239 = Delete From Array(array=w561, index=w557) -> (array with subset deleted=w563:T12)  [unwired: 1 in, 1 out]
            n240 = Reverse 1D Array(array=w562) -> (reversed array=w564:i32[])
            n241 = Reverse 1D Array(array=w563) -> (reversed array=w565:T12)
            n242 = Bundle(w564, w565) -> (w556:T13)  [unwired: 1 in]
            n243 = local write "ROI Descriptor out"(w555) -> ()
            n244 = local write "ROI Descriptor"(w556) -> ()
            n245 = property on="Image Out" class="ImageControl"("ROI"=w556) -> ()  [unwired: 2 in, 2 out]
          }
          event "Undo Button": Mouse Down {
            n246 = event-data() -> ()  [unwired: 1 in, 7 out]
            n247 = invoke on="Image Out" class="ImageControl" method="Clear ROI"() -> ()  [unwired: 3 in, 3 out]
          }
          event "Image Folder": Value Change {
            n248 = event-data() -> ()  [unwired: 1 in, 5 out]
            n249 = local read "Image File"() -> (w567:path)
            n250 = call "Vision Acquisition"("Image Path"=w567) -> ("Image Out"=w566:T2)  [unwired: 25 in, 1 out]
            n251 = local write "Image Out 2"(w566) -> ()
            n252 = local write "Image Out"(w566) -> ()
            n253 = invoke on="Image Out" class="ImageControl" method="Clear ROI"() -> ()  [unwired: 3 in, 3 out]
          }
          event "Zoom": Value Change {
            n254 = event-data() -> ()  [unwired: 1 in, 5 out]
            n255 = local read "Zoom"() -> (w568:i16)
            n256 = Bundle("Zoom"=w568, "Zoom"=w568) -> (w569:cluster{"Zoom":i16, "Zoom":i16})  [unwired: 1 in]
            n257 = property on="Image Out" class="ImageControl"("ZoomInteger"=w569) -> ()  [unwired: 2 in, 2 out]
          }
          event Timeout {
            n258 = event-data() -> ()  [unwired: 1 in, 2 out]
          }
          event "Image Out": Mouse Enter {
            (unwired) 6
            n259 = event-data() -> ()  [unwired: 1 in, 3 out]
            n260 = call "Simulate_Keyboard.vi"("Action"=0, "Virtual Key"=162) -> ()  [unwired: 7 in, 1 out]
          }
          event "Image Out": Mouse Leave {
            n261 = event-data() -> ()  [unwired: 1 in, 3 out]
            n262 = flat-sequence {
              frame #0 {
                n263 = Wait (ms)(milliseconds to wait=10) -> ()  [unwired: 1 out]
              }
              frame #1 {
                (unwired) 6
                n264 = call "Simulate_Keyboard.vi"("Action"=2, "Virtual Key"=162) -> ()  [unwired: 7 in, 1 out]
              }
            }
          }
        }
        n265 = Index Array(array=w523) -> (element=w527:T14)  [unwired: 1 in]
        n266 = Divide(x=w510, y=w487) -> (x/y=w500:sgl)
        n267 = Multiply(x=w500, y=0.5) -> (x*y=w506:dbl)
        n268 = Divide(x=w509, y=w511) -> (x/y=w499:sgl)
        n269 = Multiply(x=w499, y=0.5) -> (x*y=w505:dbl)
        n270 = Unbundle(w519) -> ("X"=w501:u32, "Y"=w502:u32)
        n271 = Subtract(x=w502, y=w505) -> (x-y=w503:dbl)
        n272 = Subtract(x=w501, y=w506) -> (x-y=w504:dbl)
        n273 = Add(x=w504, y=w500) -> (x+y=w518:dbl)
        n274 = Add(x=w503, y=w499) -> (x+y=w517:dbl)
        n275 = Build Array(w434, w457, w436, w432, w428, w458, w459, w414, w413, w406, w410, w409, w412, w397, w451, w454, w464, w455, w407, w462, w450, w444, w447, w446, w442, w440, w438) -> (w460:string[])
        n276 = local write "Current \nRecord"(w460) -> ()
        n277 = event shown="[3] \"Up Button\": Mouse Down" {
          selector: _ -> [_ _ _ _ _ _ _ _ _ _ _ _ _ _ _ _]
          dyn-events: _ -> [_ _ _ _ _ _ _ _ _ _ _ _ _ _ _ _]
          timeout: 10 -> [_ _ _ _ _ _ _ _ _ _ _ _ _ _ _ _]
          tunnel: [_ _ _ _ _ _ _ _ _ _ _ _ _ TRUE _ TRUE] -> w544
          event Timeout {
            n278 = event-data() -> ()  [unwired: 1 in, 2 out]
          }
          event "Down Button": Mouse Down {
            w912 = 0
            n279 = event-data() -> ()  [unwired: 1 in, 7 out]
            n280 = local read "NumPts 2"() -> (w879:dbl)
            n281 = local read "NumPts"() -> (w885:dbl)
            n282 = local read "Folder Index"() -> (w851:dbl)
            n283 = local read "Data File"() -> (w917:path)
            n284 = local read "Data File"() -> (w849:path)
            n285 = call "Recorded Values.vi"("Path"=w849) -> ("Recorded Char"=w847:T5, "Recorded Prop"=w846:T6, "Fabrication Prop"=w848:T7)  [unwired: 8 in]
            n286 = Unbundle By Name(w847) -> ("Mobility-Sat"=w833:dbl, "Moblitity-Lin"=w832:dbl, "On/Off"=w831:dbl, "Threshold Voltage"=w830:dbl, "Onset Voltage"=w829:dbl, "STS"=w828:dbl, "Trap Density-VT"=w827:dbl, "Trap Density-STS"=w826:dbl)
            n287 = Unbundle By Name(w848) -> ("Date Created"=w825:string, "Material"=w845:string, "Solvent"=w844:string, "Concentration"=w843:dbl, "Method"=w842:string, "Dielectric (nm)"=w841:dbl, "Treatment"=w840:string, "Comments"=w839:string)
            n288 = Unbundle By Name(w846) -> ("Date Recorded"=w838:string, "Index"=w837:string, "Length"=w836:dbl, "Width"=w835:dbl, "Sample Temp"=w834:dbl)
            n289 = local write "Rec: Material"(w845) -> ()
            n290 = local write "Date Created"(w825) -> ()
            n291 = local write "Rec: Solvent"(w844) -> ()
            n292 = local write "Rec: Concentration"(w843) -> ()
            n293 = local write "Rec: Method"(w842) -> ()
            n294 = local write "Rec: Dielectric (d)"(w841) -> ()
            n295 = local write "Surface Treatment:"(w840) -> ()
            n296 = local write "Comments"(w839) -> ()
            n297 = local write "Index"(w837) -> ()
            n298 = local write "Rec: Mobility-Sat"(w833) -> ()
            n299 = local write "Rec: Mobility-Lin"(w832) -> ()
            n300 = local write "Rec: On/Off"(w831) -> ()
            n301 = local write "Rec: VT"(w830) -> ()
            n302 = local write "Rec: Onset V"(w829) -> ()
            n303 = local write "Rec: STS"(w828) -> ()
            n304 = local write "Rec: Trap Density-VT"(w827) -> ()
            n305 = local write "Rec: Trap Density-STS"(w826) -> ()
            n306 = property on="Image Out" class="ImageControl"() -> (error out=w852:errorcluster, "Image Center Position"=w856:cluster{"X":u32, "Y":u32})  [unwired: 2 in, 1 out]
            n307 = local write "Date Recorded"(w838) -> ()
            n308 = local write "Rec: Length"(w836) -> ()
            n309 = local write "Rec: Width"(w835) -> ()
            n310 = local write "Rec: Temp"(w834) -> ()
            n311 = Strip Path(path=w917) -> (stripped path=w908:path, name=w929:string)
            n312 = local write "Data Folder"(w908) -> ()
            n313 = List Folder(path=w908) -> (filenames=w922:string[], error out=w861:errorcluster)  [unwired: 3 in, 2 out]
            n314 = Array Size(array=w922) -> (size(s)=w918:i32)
            n315 = Path To String(path=w908) -> (string=w930:string)
            n316 = Search 1D Array(1D array=w922, element=w929) -> (index of element=w919:i32)  [unwired: 1 in]
            n317 = Unbundle(w856) -> ("X"=w854:u32)  [unwired: 1 out]
            n318 = Bundle("X"=w854, 0) -> (w855:cluster{"X":u32, i32})  [unwired: 1 in]
            n319 = Decrement(x=w918) -> (x-1=w920:i32)
            n320 = Equal?(x=w919, y=w920) -> (x = y?=w921:bool)
            n321 = case shown="False" w921 {
              tunnel: w851 -> [w1057 _]
              tunnel: [w1056 0] -> w850
              frame False {
                n322 = Increment(x=w1057) -> (x+1=w1056:dbl)
              }
              frame True {
              }
            }
            n323 = Index Array(array=w922, index=w850) -> (element=w923:string)
            n324 = local write "Folder Index"(w850) -> ()
            n325 = local write "Data Name:"(w923) -> ()
            n326 = Concatenate Strings(w930, "\\", w923) -> (w928:string)
            n327 = property on="Image Out" class="ImageControl"(error in=w852, "Image Center Position"=w855) -> ()  [unwired: 1 in, 2 out]
            n328 = String To Path(string=w928) -> (path=w886:path)
            n329 = call "sub_thresh_swing_subvi.vi"("Path"=w886, "NumPts"=w879) -> ("Index"=w880:dbl, "XY Graph"=w875:cluster{dbl[], dbl[]}[], "Sub Threshold Swing"=w887:dbl)  [unwired: 9 in, 2 out]
            n330 = Decimate 1D Array(w875) -> (w878:cluster{dbl[], dbl[]}[])  [unwired: 1 out]
            n331 = Array To Cluster(array=w878) -> (cluster=w876:T8)
            n332 = Unbundle(w876) -> ("[0]"=w877:cluster{dbl[], dbl[]})  [unwired: 8 out]
            n333 = Unbundle(w877) -> (w874:dbl[], w873:dbl[])
            n334 = local write "Calc: STS"(w887) -> ()
            n335 = local write "XY Graph 2"(w875) -> ()
            n336 = local write "Index 2"(w880) -> ()
            n337 = call "mobility_subvi_07_12a_JW.vi"("Path"=w886, "NumPts"=w885) -> ("Dielectric (d)"=w889:dbl, "Index"=w894:dbl, "XY Graph"=w897:cluster{dbl[], dbl[]}[], "Length"=w888:dbl, "Vt"=w890:dbl, "Width"=w867:dbl, "Table Control"=w926:string[][], "Table Control 2"=w925:string[][], "Mobility"=w924:dbl)  [unwired: 4 in, 1 out]
            n338 = local write "Calc: VT"(w890) -> ()
            n339 = local write "New: Dielectric"(w889) -> ()
            n340 = Decimate 1D Array(w897) -> (w898:cluster{dbl[], dbl[]}[])  [unwired: 1 out]
            n341 = Array To Cluster(array=w898) -> (cluster=w900:T8)
            n342 = local write "Table Control"(w926) -> ()
            n343 = Unbundle(w900) -> ("[0]"=w899:cluster{dbl[], dbl[]})  [unwired: 8 out]
            n344 = Unbundle(w899) -> (w882:dbl[], w881:dbl[])
            n345 = local write "Calc: Mobility-Sat"(w924) -> ()
            n346 = local write "XY Graph"(w897) -> ()
            n347 = local write "Table Control 2"(w925) -> ()
            n348 = Array Subset(array=w882, index=w894, length=w885) -> (w896:dbl[])
            n349 = Array Subset(array=w881, index=w894, length=w885) -> (w895:dbl[])
            n350 = local write "Array 2"(w895) -> ()
            n351 = local write "Array"(w896) -> ()
            n352 = local write "MobVi Index"(w894) -> ()
            n353 = local write "Slide"(w894) -> ()
            n354 = Array Subset(array=w874, index=w880, length=w879) -> (w884:dbl[])
            n355 = Array Subset(array=w873, index=w880, length=w879) -> (w883:dbl[])
            n356 = local write "New: Width"(w867) -> ()
            n357 = local write "Data File"(w886) -> ()
            n358 = local write "New: Length"(w888) -> ()
            n359 = local write "Array 8"(w884) -> ()
            n360 = local write "Array 7"(w883) -> ()
            n361 = call-poly <vilib>:"Read From Spreadsheet File.vi"("file path (dialog if empty)"=w886) -> ("all rows"=w914:string[][])  [unwired: 6 in, 4 out]
            n362 = local read "Image Folder"() -> (w858:path)
            n363 = Array Size(array=w914) -> (size(s)=w913:i32[])
            n364 = List Folder(path=w858, error in=w861) -> (filenames=w907:string[], error out=w862:errorcluster)  [unwired: 2 in, 2 out]
            n365 = Index Array(array=w913, index=w912) -> (element=w892:i32)
            n366 = Subtract(x=w892, y=20) -> (x-y=w891:i32)
            n367 = property on="Slide" class="Slide (strict)"("Scale.Maximum"=w891) -> ()  [unwired: 2 in, 2 out]
            n368 = Array Subset(array=w914, index (row)=w912, index (col)=w912, length (col)=3) -> (w915:string[][])  [unwired: 1 in]
            n369 = Reshape Array(w915, w892) -> (w901:string[])
            n370 = local read "No Image"() -> (w868:path)
            n371 = Search 1D Array(1D array=w901, element="Index:") -> (index of element=w909:i32)  [unwired: 1 in]
            n372 = Increment(x=w909) -> (x+1=w910:i32)
            n373 = Index Array(array=w901, index=w910) -> (element=w860:string)
            n374 = while {
              tunnel: w907 -> [w943]
              tunnel: w860 -> [w941]
              tunnel: [w940] -> _
              tunnel: [w940] -> w906
              tunnel: w892 -> [w939]
              i -> [w940]
              stop <- w936 stop-if-true
              n375 = Index Array(array=w943, index=w940) -> (element=w944:string)
              n376 = xnode "Match Regular Expression"("input string"=w944, "regular expression"=w941) -> ("whole match"=w942:string)  [unwired: 4 in, 4 out]
              n377 = Equal?(x=w942, y=w941) -> (x = y?=w938:bool)
              n378 = Equal?(x=w939, y=w940) -> (x = y?=w937:bool)
              n379 = Or(x=w938, y=w937) -> (x .or. y?=w936:bool)
            }
            n380 = Build Path(base path=w858, name or relative path="ROI") -> (appended path=w857:path)
            n381 = Build Path(base path=w857, name or relative path=w860) -> (appended path=w866:path)
            n382 = invoke on="Image Out" class="ImageControl" method="Clear ROI"(error in=w862) -> (error out=w865:errorcluster)  [unwired: 2 in, 2 out]
            n383 = Path To String(path=w858) -> (string=w904:string)
            n384 = invoke on="Image Out" class="ImageControl" method="Clear ROI"() -> ()  [unwired: 3 in, 3 out]
            n385 = call <vilib>:"Check if File or Folder Exists.vi"("error in (no error)"=w865, "path"=w866) -> ("file or folder exists?"=w863:bool, "dup path"=w864:path)  [unwired: 7 in, 1 out]
            n386 = case shown="True" w863 {
              tunnel: w864 -> [_ w931]
              frame False {
              }
              frame True {
                n387 = Read from Text File(file (use dialog)=w931) -> (text=w935:string)  [unwired: 3 in, 3 out]
                n388 = property on="Image Out" class="ImageControl"() -> ("ROI"=w932:T9)  [unwired: 2 in, 2 out]
                n389 = Unflatten From String(type=w932, binary string=w935) -> (value=w933:T9, error out=w934:errorcluster)  [unwired: 3 in, 1 out]
                n390 = property on="Image Out" class="ImageControl"(error in=w934, "ROI"=w933) -> ()  [unwired: 1 in, 2 out]
              }
            }
            n391 = Index Array(array=w907, index=w906) -> (element=w871:string)
            n392 = Empty String/Path?(string/path=w871) -> (empty?=w872:bool)
            n393 = Concatenate Strings(w904, "\\", w871) -> (w903:string)
            n394 = String To Path(string=w903) -> (path=w870:path)
            n395 = Select(t=w868, s=w872, f=w870) -> (s? t:f=w869:path)
            n396 = call "Vision Acquisition4"("Image Path"=w869) -> ("Image Out"=w905:T2)  [unwired: 25 in, 1 out]
            n397 = local write "Image File"(w869) -> ()
            n398 = local write "Image Out 2"(w905) -> ()
            n399 = local write "Image Out"(w905) -> ()
            n400 = local write "Image Name"(w871) -> ()
          }
          event "Data File": Value Change {
            w1146 = 0
            n401 = event-data() -> ()  [unwired: 1 in, 5 out]
            n402 = local read "Data File"() -> (w1083:path)
            n403 = call "Recorded Values.vi"("Path"=w1083) -> ("Recorded Char"=w1081:T5, "Recorded Prop"=w1080:T6, "Fabrication Prop"=w1082:T7)  [unwired: 8 in]
            n404 = Unbundle By Name(w1081) -> ("Mobility-Sat"=w1067:dbl, "Moblitity-Lin"=w1066:dbl, "On/Off"=w1065:dbl, "Threshold Voltage"=w1064:dbl, "Onset Voltage"=w1063:dbl, "STS"=w1062:dbl, "Trap Density-VT"=w1061:dbl, "Trap Density-STS"=w1060:dbl)
            n405 = Unbundle By Name(w1082) -> ("Date Created"=w1059:string, "Material"=w1079:string, "Solvent"=w1078:string, "Concentration"=w1077:dbl, "Method"=w1076:string, "Dielectric (nm)"=w1075:dbl, "Treatment"=w1074:string, "Comments"=w1073:string)
            n406 = Unbundle By Name(w1080) -> ("Date Recorded"=w1072:string, "Index"=w1071:string, "Length"=w1070:dbl, "Width"=w1069:dbl, "Sample Temp"=w1068:dbl)
            n407 = local write "Date Created"(w1059) -> ()
            n408 = local write "Rec: Material"(w1079) -> ()
            n409 = local read "NumPts"() -> (w1119:dbl)
            n410 = local read "Data File"() -> (w1142:path)
            n411 = local write "Rec: Solvent"(w1078) -> ()
            n412 = local write "Rec: Concentration"(w1077) -> ()
            n413 = local write "Rec: Method"(w1076) -> ()
            n414 = local write "Rec: Dielectric (d)"(w1075) -> ()
            n415 = local write "Surface Treatment:"(w1074) -> ()
            n416 = local write "Comments"(w1073) -> ()
            n417 = local write "Index"(w1071) -> ()
            n418 = local write "Rec: Mobility-Sat"(w1067) -> ()
            n419 = local write "Rec: Mobility-Lin"(w1066) -> ()
            n420 = local write "Rec: On/Off"(w1065) -> ()
            n421 = local write "Rec: VT"(w1064) -> ()
            n422 = local write "Rec: Onset V"(w1063) -> ()
            n423 = local write "Rec: STS"(w1062) -> ()
            n424 = local write "Rec: Trap Density-VT"(w1061) -> ()
            n425 = local write "Rec: Trap Density-STS"(w1060) -> ()
            n426 = local write "Date Recorded"(w1072) -> ()
            n427 = local write "Rec: Length"(w1070) -> ()
            n428 = local write "Rec: Width"(w1069) -> ()
            n429 = local write "Rec: Temp"(w1068) -> ()
            n430 = local read "NumPts 2"() -> (w1113:dbl)
            n431 = property on="Image Out" class="ImageControl"() -> (error out=w1085:errorcluster, "Image Center Position"=w1089:cluster{"X":u32, "Y":u32})  [unwired: 2 in, 1 out]
            n432 = Strip Path(path=w1142) -> (stripped path=w1141:path, name=w1158:string)
            n433 = local write "Data Folder"(w1141) -> ()
            n434 = List Folder(path=w1141) -> (filenames=w1151:string[], error out=w1095:errorcluster)  [unwired: 3 in, 2 out]
            n435 = Unbundle(w1089) -> ("X"=w1087:u32)  [unwired: 1 out]
            n436 = Path To String(path=w1141) -> (string=w1159:string)
            n437 = Search 1D Array(1D array=w1151, element=w1158) -> (index of element=w1084:i32)  [unwired: 1 in]
            n438 = Index Array(array=w1151, index=w1084) -> (element=w1152:string)
            n439 = Bundle("X"=w1087, 0) -> (w1088:cluster{"X":u32, i32})  [unwired: 1 in]
            n440 = local write "Data Name:"(w1152) -> ()
            n441 = property on="Image Out" class="ImageControl"(error in=w1085, "Image Center Position"=w1088) -> ()  [unwired: 1 in, 2 out]
            n442 = local write "Folder Index"(w1084) -> ()
            n443 = Concatenate Strings(w1159, "\\", w1152) -> (w1157:string)
            n444 = String To Path(string=w1157) -> (path=w1120:path)
            n445 = call "sub_thresh_swing_subvi.vi"("Path"=w1120, "NumPts"=w1113) -> ("Index"=w1114:dbl, "XY Graph"=w1109:cluster{dbl[], dbl[]}[], "Sub Threshold Swing"=w1118:dbl)  [unwired: 9 in, 2 out]
            n446 = Decimate 1D Array(w1109) -> (w1112:cluster{dbl[], dbl[]}[])  [unwired: 1 out]
            n447 = Array To Cluster(array=w1112) -> (cluster=w1110:T8)
            n448 = Unbundle(w1110) -> ("[0]"=w1111:cluster{dbl[], dbl[]})  [unwired: 8 out]
            n449 = Unbundle(w1111) -> (w1107:dbl[], w1106:dbl[])
            n450 = local write "Index 2"(w1114) -> ()
            n451 = call "mobility_subvi_07_12a_JW.vi"("Path"=w1120, "NumPts"=w1119) -> ("Dielectric (d)"=w1122:dbl, "Index"=w1127:dbl, "XY Graph"=w1130:cluster{dbl[], dbl[]}[], "Length"=w1121:dbl, "Vt"=w1123:dbl, "Width"=w1100:dbl, "Table Control"=w1155:string[][], "Table Control 2"=w1154:string[][], "Mobility"=w1153:dbl)  [unwired: 4 in, 1 out]
            n452 = local write "Rec: Dielectric (d)"(w1122) -> ()
            n453 = local write "New: Dielectric"(w1122) -> ()
            n454 = Decimate 1D Array(w1130) -> (w1131:cluster{dbl[], dbl[]}[])  [unwired: 1 out]
            n455 = local write "Table Control"(w1155) -> ()
            n456 = Array To Cluster(array=w1131) -> (cluster=w1133:T8)
            n457 = Unbundle(w1133) -> ("[0]"=w1132:cluster{dbl[], dbl[]})  [unwired: 8 out]
            n458 = local write "Calc: VT"(w1123) -> ()
            n459 = local write "Calc: STS"(w1118) -> ()
            n460 = local write "Calc: Mobility-Sat"(w1153) -> ()
            n461 = Unbundle(w1132) -> (w1108:dbl[], w1115:dbl[])
            n462 = local write "XY Graph"(w1130) -> ()
            n463 = local write "Table Control 2"(w1154) -> ()
            n464 = local write "XY Graph 2"(w1109) -> ()
            n465 = Array Subset(array=w1107, index=w1114, length=w1113) -> (w1117:dbl[])
            n466 = Array Subset(array=w1106, index=w1114, length=w1113) -> (w1116:dbl[])
            n467 = local write "New: Length"(w1121) -> ()
            n468 = local write "MobVi Index"(w1127) -> ()
            n469 = Array Subset(array=w1108, index=w1127, length=w1119) -> (w1129:dbl[])
            n470 = Array Subset(array=w1115, index=w1127, length=w1119) -> (w1128:dbl[])
            n471 = local write "Array 8"(w1117) -> ()
            n472 = local write "Array 7"(w1116) -> ()
            n473 = local write "New: Width"(w1100) -> ()
            n474 = local write "Array 2"(w1128) -> ()
            n475 = local write "Array"(w1129) -> ()
            n476 = local write "Data File"(w1120) -> ()
            n477 = local read "Image Folder"() -> (w1091:path)
            n478 = local write "Slide"(w1127) -> ()
            n479 = List Folder(path=w1091, error in=w1095) -> (filenames=w1139:string[], error out=w1094:errorcluster)  [unwired: 2 in, 2 out]
            n480 = call-poly <vilib>:"Read From Spreadsheet File.vi"("file path (dialog if empty)"=w1120) -> ("all rows"=w1148:string[][])  [unwired: 6 in, 4 out]
            n481 = Array Size(array=w1148) -> (size(s)=w1147:i32[])
            n482 = Index Array(array=w1147, index=w1146) -> (element=w1126:i32)
            n483 = Subtract(x=w1126, y=20) -> (x-y=w1124:i32)
            n484 = property on="Slide" class="Slide (strict)"("Scale.Maximum"=w1124) -> ()  [unwired: 2 in, 2 out]
            n485 = Array Subset(array=w1148, index (row)=w1146, index (col)=w1146, length (col)=3) -> (w1149:string[][])  [unwired: 1 in]
            n486 = Reshape Array(w1149, w1126) -> (w1134:string[])
            n487 = Search 1D Array(1D array=w1134, element="Index:") -> (index of element=w1143:i32)  [unwired: 1 in]
            n488 = Increment(x=w1143) -> (x+1=w1144:i32)
            n489 = Index Array(array=w1134, index=w1144) -> (element=w1093:string)
            n490 = while {
              tunnel: w1139 -> [w1172]
              tunnel: w1093 -> [w1170]
              tunnel: [w1169] -> _
              tunnel: [w1169] -> w1138
              tunnel: w1126 -> [w1168]
              i -> [w1169]
              stop <- w1165 stop-if-true
              n491 = Index Array(array=w1172, index=w1169) -> (element=w1173:string)
              n492 = xnode "Match Regular Expression"("input string"=w1173, "regular expression"=w1170) -> ("whole match"=w1171:string)  [unwired: 4 in, 4 out]
              n493 = Equal?(x=w1171, y=w1170) -> (x = y?=w1167:bool)
              n494 = Equal?(x=w1168, y=w1169) -> (x = y?=w1166:bool)
              n495 = Or(x=w1167, y=w1166) -> (x .or. y?=w1165:bool)
            }
            n496 = local write "Index"(w1093) -> ()
            n497 = Build Path(base path=w1091, name or relative path="ROI") -> (appended path=w1090:path)
            n498 = Path To String(path=w1091) -> (string=w1137:string)
            n499 = local read "No Image"() -> (w1101:path)
            n500 = Build Path(base path=w1090, name or relative path=w1093) -> (appended path=w1099:path)
            n501 = invoke on="Image Out" class="ImageControl" method="Clear ROI"(error in=w1094) -> (error out=w1098:errorcluster)  [unwired: 2 in, 2 out]
            n502 = Index Array(array=w1139, index=w1138) -> (element=w1104:string)
            n503 = Empty String/Path?(string/path=w1104) -> (empty?=w1105:bool)
            n504 = Concatenate Strings(w1137, "\\", w1104) -> (w1136:string)
            n505 = String To Path(string=w1136) -> (path=w1103:path)
            n506 = Select(t=w1101, s=w1105, f=w1103) -> (s? t:f=w1102:path)
            n507 = call "Vision Acquisition3"("Image Path"=w1102) -> ("Image Out"=w1140:T2)  [unwired: 25 in, 1 out]
            n508 = local write "Image File"(w1102) -> ()
            n509 = local write "Image Out 2"(w1140) -> ()
            n510 = local write "Image Out"(w1140) -> ()
            n511 = local write "Image Name"(w1104) -> ()
            n512 = call <vilib>:"Check if File or Folder Exists.vi"("error in (no error)"=w1098, "path"=w1099) -> ("file or folder exists?"=w1096:bool, "dup path"=w1097:path)  [unwired: 7 in, 1 out]
            n513 = invoke on="Image Out" class="ImageControl" method="Clear ROI"() -> ()  [unwired: 3 in, 3 out]
            n514 = case shown="True" w1096 {
              tunnel: w1097 -> [_ w1160]
              frame False {
              }
              frame True {
                n515 = Read from Text File(file (use dialog)=w1160) -> (text=w1164:string)  [unwired: 3 in, 3 out]
                n516 = property on="Image Out" class="ImageControl"() -> ("ROI"=w1161:T9)  [unwired: 2 in, 2 out]
                n517 = Unflatten From String(type=w1161, binary string=w1164) -> (value=w1162:T9, error out=w1163:errorcluster)  [unwired: 3 in, 1 out]
                n518 = property on="Image Out" class="ImageControl"(error in=w1163, "ROI"=w1162) -> ()  [unwired: 1 in, 2 out]
              }
            }
          }
          event "Up Button": Mouse Down {
            w1374 = 0
            n519 = event-data() -> ()  [unwired: 1 in, 5 out]
            n520 = local read "Data File"() -> (w1309:path)
            n521 = call "Recorded Values.vi"("Path"=w1309) -> ("Recorded Char"=w1307:T5, "Recorded Prop"=w1306:T6, "Fabrication Prop"=w1308:T7)  [unwired: 8 in]
            n522 = Unbundle By Name(w1307) -> ("Mobility-Sat"=w1293:dbl, "Moblitity-Lin"=w1292:dbl, "On/Off"=w1291:dbl, "Threshold Voltage"=w1290:dbl, "Onset Voltage"=w1289:dbl, "STS"=w1288:dbl, "Trap Density-VT"=w1287:dbl, "Trap Density-STS"=w1286:dbl)
            n523 = Unbundle By Name(w1308) -> ("Date Created"=w1285:string, "Material"=w1305:string, "Solvent"=w1304:string, "Concentration"=w1303:dbl, "Method"=w1302:string, "Dielectric (nm)"=w1301:dbl, "Treatment"=w1300:string, "Comments"=w1299:string)
            n524 = Unbundle By Name(w1306) -> ("Date Recorded"=w1298:string, "Index"=w1297:string, "Length"=w1296:dbl, "Width"=w1295:dbl, "Sample Temp"=w1294:dbl)
            n525 = local read "Data File"() -> (w1370:path)
            n526 = local read "NumPts 2"() -> (w1345:dbl)
            n527 = local write "Date Created"(w1285) -> ()
            n528 = local write "Rec: Material"(w1305) -> ()
            n529 = local write "Rec: Solvent"(w1304) -> ()
            n530 = local write "Rec: Concentration"(w1303) -> ()
            n531 = local write "Rec: Method"(w1302) -> ()
            n532 = local write "Rec: Dielectric (d)"(w1301) -> ()
            n533 = local write "Surface Treatment:"(w1300) -> ()
            n534 = local write "Comments"(w1299) -> ()
            n535 = local write "Index"(w1297) -> ()
            n536 = local write "Rec: Mobility-Sat"(w1293) -> ()
            n537 = local write "Rec: Mobility-Lin"(w1292) -> ()
            n538 = local write "Rec: On/Off"(w1291) -> ()
            n539 = local write "Rec: VT"(w1290) -> ()
            n540 = local write "Rec: Onset V"(w1289) -> ()
            n541 = local write "Rec: STS"(w1288) -> ()
            n542 = local write "Rec: Trap Density-VT"(w1287) -> ()
            n543 = local write "Rec: Trap Density-STS"(w1286) -> ()
            n544 = local read "NumPts"() -> (w1350:dbl)
            n545 = local write "Date Recorded"(w1298) -> ()
            n546 = local write "Rec: Length"(w1296) -> ()
            n547 = local write "Rec: Width"(w1295) -> ()
            n548 = local write "Rec: Temp"(w1294) -> ()
            n549 = local read "Folder Index"() -> (w1311:dbl)
            n550 = property on="Image Out" class="ImageControl"() -> (error out=w1314:errorcluster, "Image Center Position"=w1318:cluster{"X":u32, "Y":u32})  [unwired: 2 in, 1 out]
            n551 = Strip Path(path=w1370) -> (stripped path=w1369:path, name=w1388:string)
            n552 = local write "Data Folder"(w1369) -> ()
            n553 = List Folder(path=w1369) -> (filenames=w1379:string[], error out=w1324:errorcluster)  [unwired: 3 in, 2 out]
            n554 = Path To String(path=w1369) -> (string=w1389:string)
            n555 = Search 1D Array(1D array=w1379, element=w1388) -> (index of element=w1380:i32)  [unwired: 1 in]
            n556 = Unbundle(w1318) -> ("X"=w1316:u32)  [unwired: 1 out]
            n557 = Equal To 0?(x=w1380) -> (x = 0?=w1381:bool)
            n558 = Bundle("X"=w1316, 0) -> (w1317:cluster{"X":u32, i32})  [unwired: 1 in]
            n559 = property on="Image Out" class="ImageControl"(error in=w1314, "Image Center Position"=w1317) -> ()  [unwired: 1 in, 2 out]
            n560 = Array Size(array=w1379) -> (size(s)=w1312:i32)
            n561 = case shown="True" w1381 {
              tunnel: w1311 -> [w1516 _]
              tunnel: [w1515 w1517] -> w1310
              tunnel: w1312 -> [_ w1518]
              frame False {
                n562 = Decrement(x=w1516) -> (x-1=w1515:dbl)
              }
              frame True {
                n563 = Decrement(x=w1518) -> (x-1=w1517:i32)
              }
            }
            n564 = Index Array(array=w1379, index=w1310) -> (element=w1382:string)
            n565 = local write "Data Name:"(w1382) -> ()
            n566 = local write "Folder Index"(w1310) -> ()
            n567 = Concatenate Strings(w1389, "\\", w1382) -> (w1387:string)
            n568 = String To Path(string=w1387) -> (path=w1351:path)
            n569 = call "sub_thresh_swing_subvi.vi"("Path"=w1351, "NumPts"=w1345) -> ("Index"=w1344:dbl, "XY Graph"=w1340:cluster{dbl[], dbl[]}[], "Sub Threshold Swing"=w1352:dbl)  [unwired: 9 in, 2 out]
            n570 = Decimate 1D Array(w1340) -> (w1343:cluster{dbl[], dbl[]}[])  [unwired: 1 out]
            n571 = Array To Cluster(array=w1343) -> (cluster=w1341:T8)
            n572 = Unbundle(w1341) -> ("[0]"=w1342:cluster{dbl[], dbl[]})  [unwired: 8 out]
            n573 = Unbundle(w1342) -> (w1339:dbl[], w1338:dbl[])
            n574 = Array Subset(array=w1339, index=w1344, length=w1345) -> (w1347:dbl[])
            n575 = Array Subset(array=w1338, index=w1344, length=w1345) -> (w1346:dbl[])
            n576 = local write "Calc: STS"(w1352) -> ()
            n577 = local write "Array 8"(w1347) -> ()
            n578 = local write "Array 7"(w1346) -> ()
            n579 = call "mobility_subvi_07_12a_JW.vi"("Path"=w1351, "NumPts"=w1350) -> ("Dielectric (d)"=w1354:dbl, "Index"=w1356:dbl, "XY Graph"=w1362:cluster{dbl[], dbl[]}[], "Length"=w1353:dbl, "Vt"=w1355:dbl, "Width"=w1335:dbl, "Table Control"=w1385:string[][], "Table Control 2"=w1384:string[][], "Mobility"=w1383:dbl)  [unwired: 4 in, 1 out]
            n580 = local write "New: Length"(w1353) -> ()
            n581 = local write "New: Dielectric"(w1354) -> ()
            n582 = local write "New: Width"(w1335) -> ()
            n583 = local write "Table Control"(w1385) -> ()
            n584 = Decimate 1D Array(w1362) -> (w1363:cluster{dbl[], dbl[]}[])  [unwired: 1 out]
            n585 = local write "XY Graph 2"(w1340) -> ()
            n586 = local write "Calc: Mobility-Sat"(w1383) -> ()
            n587 = Array To Cluster(array=w1363) -> (cluster=w1365:T8)
            n588 = local write "XY Graph"(w1362) -> ()
            n589 = local write "Index 2"(w1344) -> ()
            n590 = local write "Table Control 2"(w1384) -> ()
            n591 = Unbundle(w1365) -> ("[0]"=w1364:cluster{dbl[], dbl[]})  [unwired: 8 out]
            n592 = Unbundle(w1364) -> (w1349:dbl[], w1348:dbl[])
            n593 = local write "Calc: VT"(w1355) -> ()
            n594 = Array Subset(array=w1349, index=w1356, length=w1350) -> (w1361:dbl[])
            n595 = Array Subset(array=w1348, index=w1356, length=w1350) -> (w1360:dbl[])
            n596 = local write "Array 2"(w1360) -> ()
            n597 = local write "Array"(w1361) -> ()
            n598 = local write "MobVi Index"(w1356) -> ()
            n599 = local write "Data File"(w1351) -> ()
            n600 = local read "Image Folder"() -> (w1313:path)
            n601 = local write "Slide"(w1356) -> ()
            n602 = List Folder(path=w1313, error in=w1324) -> (filenames=w1368:string[], error out=w1323:errorcluster)  [unwired: 2 in, 2 out]
            n603 = call-poly <vilib>:"Read From Spreadsheet File.vi"("file path (dialog if empty)"=w1351) -> ("all rows"=w1376:string[][])  [unwired: 6 in, 4 out]
            n604 = Array Size(array=w1376) -> (size(s)=w1375:i32[])
            n605 = Index Array(array=w1375, index=w1374) -> (element=w1358:i32)
            n606 = Subtract(x=w1358, y=20) -> (x-y=w1357:i32)
            n607 = property on="Slide" class="Slide (strict)"("Scale.Maximum"=w1357) -> ()  [unwired: 2 in, 2 out]
            n608 = Array Subset(array=w1376, index (row)=w1374, index (col)=w1374, length (col)=3) -> (w1377:string[][])  [unwired: 1 in]
            n609 = Reshape Array(w1377, w1358) -> (w1366:string[])
            n610 = Search 1D Array(1D array=w1366, element="Index:") -> (index of element=w1371:i32)  [unwired: 1 in]
            n611 = Increment(x=w1371) -> (x+1=w1372:i32)
            n612 = Index Array(array=w1366, index=w1372) -> (element=w1320:string)
            n613 = while {
              tunnel: w1368 -> [w1402]
              tunnel: w1320 -> [w1400]
              tunnel: [w1399] -> w1367
              tunnel: w1358 -> [w1398]
              i -> [w1399]
              stop <- w1395 stop-if-true
              n614 = Index Array(array=w1402, index=w1399) -> (element=w1403:string)
              n615 = xnode "Match Regular Expression"("input string"=w1403, "regular expression"=w1400) -> ("whole match"=w1401:string)  [unwired: 4 in, 4 out]
              n616 = Equal?(x=w1401, y=w1400) -> (x = y?=w1397:bool)
              n617 = Equal?(x=w1398, y=w1399) -> (x = y?=w1396:bool)
              n618 = Or(x=w1397, y=w1396) -> (x .or. y?=w1395:bool)
            }
            n619 = local write "Index"(w1320) -> ()
            n620 = Build Path(base path=w1313, name or relative path="ROI") -> (appended path=w1321:path)
            n621 = Build Path(base path=w1321, name or relative path=w1320) -> (appended path=w1319:path)
            n622 = invoke on="Image Out" class="ImageControl" method="Clear ROI"(error in=w1323) -> (error out=w1327:errorcluster)  [unwired: 2 in, 2 out]
            n623 = call <vilib>:"Check if File or Folder Exists.vi"("error in (no error)"=w1327, "path"=w1319) -> ("file or folder exists?"=w1325:bool, "dup path"=w1326:path)  [unwired: 7 in, 1 out]
            n624 = local read "No Image"() -> (w1336:path)
            n625 = Index Array(array=w1368, index=w1367) -> (element=w1329:string)
            n626 = Build Path(base path=w1313, name or relative path=w1329) -> (appended path=w1328:path)
            n627 = local write "Image Name"(w1329) -> ()
            n628 = case shown="True" w1325 {
              tunnel: w1326 -> [_ w1390]
              frame False {
              }
              frame True {
                n629 = Read from Text File(file (use dialog)=w1390) -> (text=w1394:string)  [unwired: 3 in, 3 out]
                n630 = property on="Image Out" class="ImageControl"() -> ("ROI"=w1391:T9)  [unwired: 2 in, 2 out]
                n631 = Unflatten From String(type=w1391, binary string=w1394) -> (value=w1392:T9, error out=w1393:errorcluster)  [unwired: 3 in, 1 out]
                n632 = property on="Image Out" class="ImageControl"(error in=w1393, "ROI"=w1392) -> ()  [unwired: 1 in, 2 out]
              }
            }
            n633 = Empty String/Path?(string/path=w1329) -> (empty?=w1337:bool)
            n634 = Select(t=w1336, s=w1337, f=w1328) -> (s? t:f=w1330:path)
            n635 = call "Vision Acquisition5"("Image Path"=w1330) -> ("Image Out"=w1334:T2)  [unwired: 25 in, 1 out]
            n636 = local write "Image File"(w1330) -> ()
            n637 = local write "Image Out 2"(w1334) -> ()
            n638 = local write "Image Out"(w1334) -> ()
            n639 = call <vilib>:"Get File Extension.vi"("file"=w1330) -> ("lowercase file extension"=w1332:string)  [unwired: 7 in, 3 out]
            n640 = local write "String"(w1332) -> ()
            n641 = Search 1D Array(1D array=string[] ["bmp", "jpeg", "png", "jpg", "gif"], element=w1332) -> (index of element=w1331:i32)  [unwired: 1 in]
            n642 = Less Than 0?(x=w1331) -> ()  [unwired: 1 out]
          }
          event "Save Changes? 3": Mouse Down {
            n643 = event-data() -> ()  [unwired: 1 in, 7 out]
            n644 = local read "Image Folder"() -> (w1519:path)
            n645 = Build Path(base path=w1519, name or relative path="ROI") -> (appended path=w1526:path)
            n646 = call <vilib>:"Check if File or Folder Exists.vi"("path"=w1526) -> ("file or folder exists?"=w1528:bool, "dup path"=w1525:path)  [unwired: 8 in, 1 out]
            n647 = case shown="False" w1528 {
              tunnel: w1525 -> [w1530 w1531]
              tunnel: [w1529 w1531] -> w1520
              frame False {
                n648 = Create Folder(path (use dialog)=w1530) -> (created path=w1529:path)  [unwired: 2 in, 2 out]
              }
              frame True {
              }
            }
            n649 = property on="Image Out" class="ImageControl"() -> ("ROI"=w1524:T9)  [unwired: 2 in, 2 out]
            n650 = local read "Index"() -> (w1522:string)
            n651 = Flatten To String(anything=w1524) -> (data string=w1523:string)  [unwired: 3 in, 2 out]
            n652 = Build Path(base path=w1520, name or relative path=w1522) -> (appended path=w1521:path)
            n653 = Write to Text File(file (use dialog)=w1521, text=w1523) -> ()  [unwired: 2 in, 3 out]
          }
          event "Next Button": Mouse Down {
            n654 = event-data() -> ()  [unwired: 1 in, 5 out]
            n655 = local read "XY Graph"() -> (w1544:cluster{dbl[], dbl[]}[])
            n656 = local read "MobVi Index"() -> (w1546:dbl)
            n657 = local read "NumPts"() -> (w1545:dbl)
            n658 = Decimate 1D Array(w1544) -> (w1540:cluster{dbl[], dbl[]}[], w1539:cluster{dbl[], dbl[]}[])
            n659 = Array To Cluster(array=w1540) -> (cluster=w1550:T8)
            n660 = Unbundle(w1550) -> ("[0]"=w1549:cluster{dbl[], dbl[]})  [unwired: 8 out]
            n661 = Increment(x=w1546) -> (x+1=w1541:dbl)
            n662 = Unbundle(w1549) -> (w1548:dbl[], w1547:dbl[])
            n663 = local write "MobVi Index"(w1541) -> ()
            n664 = Array Subset(array=w1548, index=w1541, length=w1545) -> (w1537:dbl[])
            n665 = Array Subset(array=w1547, index=w1541, length=w1545) -> (w1536:dbl[])
            n666 = Bundle(w1537, w1536) -> (w1543:cluster{dbl[], dbl[]})  [unwired: 1 in]
            n667 = Build Array (concatenate)(w1540, w1539, w1543) -> (w1542:cluster{dbl[], dbl[]}[])
            n668 = local write "XY Graph"(w1542) -> ()
            n669 = local read "New: Dielectric"() -> (w1535:dbl)
            n670 = local write "Array 2"(w1536) -> ()
            n671 = local read "New: Length"() -> (w1534:dbl)
            n672 = local write "Array"(w1537) -> ()
            n673 = local read "New: Width"() -> (w1533:dbl)
            n674 = call "mob_calc_subvi.vi"("Width"=w1533, "Length"=w1534, "Dielectric (d)"=w1535, "Array 2"=w1536, "Array"=w1537) -> ("Vt"=w1532:dbl, "Mobility"=w1538:dbl)  [unwired: 4 in, 1 out]
            n675 = local write "New: Mobility-Sat"(w1538) -> ()
            n676 = local write "New: VT"(w1532) -> ()
          }
          event "Next Button 2": Mouse Down {
            n677 = event-data() -> ()  [unwired: 1 in, 7 out]
            n678 = local read "XY Graph 2"() -> (w1559:cluster{dbl[], dbl[]}[])
            n679 = local read "Index 2"() -> (w1561:dbl)
            n680 = local read "NumPts 2"() -> (w1560:dbl)
            n681 = Decimate 1D Array(w1559) -> (w1555:cluster{dbl[], dbl[]}[], w1554:cluster{dbl[], dbl[]}[])
            n682 = Array To Cluster(array=w1555) -> (cluster=w1565:T8)
            n683 = Unbundle(w1565) -> ("[0]"=w1564:cluster{dbl[], dbl[]})  [unwired: 8 out]
            n684 = Increment(x=w1561) -> (x+1=w1556:dbl)
            n685 = Unbundle(w1564) -> (w1563:dbl[], w1562:dbl[])
            n686 = local write "Index 2"(w1556) -> ()
            n687 = Array Subset(array=w1563, index=w1556, length=w1560) -> (w1552:dbl[])
            n688 = Array Subset(array=w1562, index=w1556, length=w1560) -> (w1551:dbl[])
            n689 = Bundle(w1552, w1551) -> (w1558:cluster{dbl[], dbl[]})  [unwired: 1 in]
            n690 = Build Array (concatenate)(w1555, w1554, w1558) -> (w1557:cluster{dbl[], dbl[]}[])
            n691 = local write "XY Graph 2"(w1557) -> ()
            n692 = local write "Array 8"(w1552) -> ()
            n693 = call "sts_calc_subvi.vi"("Array 2"=w1552, "Array"=w1551) -> ("STS"=w1553:dbl)  [unwired: 9 in]
            n694 = local write "Array 7"(w1551) -> ()
            n695 = local write "New: STS"(w1553) -> ()
          }
          event "Previous Button 2": Mouse Down {
            n696 = event-data() -> ()  [unwired: 1 in, 7 out]
            n697 = local read "XY Graph 2"() -> (w1575:cluster{dbl[], dbl[]}[])
            n698 = local read "NumPts 2"() -> (w1576:dbl)
            n699 = local read "Index 2"() -> (w1568:dbl)
            n700 = Decimate 1D Array(w1575) -> (w1572:cluster{dbl[], dbl[]}[], w1571:cluster{dbl[], dbl[]}[])
            n701 = Array To Cluster(array=w1572) -> (cluster=w1580:T8)
            n702 = Unbundle(w1580) -> ("[0]"=w1579:cluster{dbl[], dbl[]})  [unwired: 8 out]
            n703 = Decrement(x=w1568) -> (x-1=w1569:dbl)
            n704 = Unbundle(w1579) -> (w1578:dbl[], w1577:dbl[])
            n705 = local write "Index 2"(w1569) -> ()
            n706 = Array Subset(array=w1578, index=w1569, length=w1576) -> (w1566:dbl[])
            n707 = Array Subset(array=w1577, index=w1569, length=w1576) -> (w1567:dbl[])
            n708 = Bundle(w1566, w1567) -> (w1574:cluster{dbl[], dbl[]})  [unwired: 1 in]
            n709 = Build Array (concatenate)(w1572, w1571, w1574) -> (w1573:cluster{dbl[], dbl[]}[])
            n710 = local write "XY Graph 2"(w1573) -> ()
            n711 = local write "Array 7"(w1567) -> ()
            n712 = call "sts_calc_subvi.vi"("Array 2"=w1566, "Array"=w1567) -> ("STS"=w1570:dbl)  [unwired: 9 in]
            n713 = local write "Array 8"(w1566) -> ()
            n714 = local write "New: STS"(w1570) -> ()
          }
          event "Previous Button": Mouse Down {
            n715 = event-data() -> ()  [unwired: 1 in, 5 out]
            n716 = local read "XY Graph"() -> (w1594:cluster{dbl[], dbl[]}[])
            n717 = Decimate 1D Array(w1594) -> (w1591:cluster{dbl[], dbl[]}[], w1590:cluster{dbl[], dbl[]}[])
            n718 = local read "MobVi Index"() -> (w1589:dbl)
            n719 = local read "NumPts"() -> (w1595:dbl)
            n720 = Array To Cluster(array=w1591) -> (cluster=w1599:T8)
            n721 = Unbundle(w1599) -> ("[0]"=w1598:cluster{dbl[], dbl[]})  [unwired: 8 out]
            n722 = Decrement(x=w1589) -> (x-1=w1588:dbl)
            n723 = Unbundle(w1598) -> (w1597:dbl[], w1596:dbl[])
            n724 = local read "New: Dielectric"() -> (w1582:dbl)
            n725 = Array Subset(array=w1597, index=w1588, length=w1595) -> (w1587:dbl[])
            n726 = local write "MobVi Index"(w1588) -> ()
            n727 = Array Subset(array=w1596, index=w1588, length=w1595) -> (w1586:dbl[])
            n728 = Bundle(w1587, w1586) -> (w1593:cluster{dbl[], dbl[]})  [unwired: 1 in]
            n729 = Build Array (concatenate)(w1591, w1590, w1593) -> (w1592:cluster{dbl[], dbl[]}[])
            n730 = local write "XY Graph"(w1592) -> ()
            n731 = local read "New: Length"() -> (w1583:dbl)
            n732 = local write "Array 2"(w1586) -> ()
            n733 = local read "New: Width"() -> (w1584:dbl)
            n734 = call "mob_calc_subvi.vi"("Width"=w1584, "Length"=w1583, "Dielectric (d)"=w1582, "Array 2"=w1586, "Array"=w1587) -> ("Vt"=w1581:dbl, "Mobility"=w1585:dbl)  [unwired: 4 in, 1 out]
            n735 = local write "New: Mobility-Sat"(w1585) -> ()
            n736 = local write "Array"(w1587) -> ()
            n737 = local write "New: VT"(w1581) -> ()
          }
          event "Slide": Value Change {
            n738 = event-data() -> ()  [unwired: 1 in, 5 out]
            n739 = local read "XY Graph"() -> (w1612:cluster{dbl[], dbl[]}[])
            n740 = local read "Slide"() -> (w1601:dbl)
            n741 = Decimate 1D Array(w1612) -> (w1609:cluster{dbl[], dbl[]}[], w1608:cluster{dbl[], dbl[]}[])
            n742 = local read "NumPts"() -> (w1613:dbl)
            n743 = Array To Cluster(array=w1609) -> (cluster=w1617:T8)
            n744 = Unbundle(w1617) -> ("[0]"=w1616:cluster{dbl[], dbl[]})  [unwired: 8 out]
            n745 = Unbundle(w1616) -> (w1615:dbl[], w1614:dbl[])
            n746 = local read "New: Dielectric"() -> (w1602:dbl)
            n747 = Array Subset(array=w1615, index=w1601, length=w1613) -> (w1607:dbl[])
            n748 = local write "MobVi Index"(w1601) -> ()
            n749 = Array Subset(array=w1614, index=w1601, length=w1613) -> (w1606:dbl[])
            n750 = Bundle(w1607, w1606) -> (w1611:cluster{dbl[], dbl[]})  [unwired: 1 in]
            n751 = Build Array (concatenate)(w1609, w1608, w1611) -> (w1610:cluster{dbl[], dbl[]}[])
            n752 = local write "XY Graph"(w1610) -> ()
            n753 = local read "New: Length"() -> (w1603:dbl)
            n754 = local write "Array 2"(w1606) -> ()
            n755 = local read "New: Width"() -> (w1604:dbl)
            n756 = call "mob_calc_subvi.vi"("Width"=w1604, "Length"=w1603, "Dielectric (d)"=w1602, "Array 2"=w1606, "Array"=w1607) -> ("Vt"=w1600:dbl, "Mobility"=w1605:dbl)  [unwired: 4 in, 1 out]
            n757 = local write "New: Mobility-Sat"(w1605) -> ()
            n758 = local write "Array"(w1607) -> ()
            n759 = local write "New: VT"(w1600) -> ()
          }
          event "Slide 2": Value Change {
            n760 = event-data() -> ()  [unwired: 1 in, 5 out]
            n761 = local read "XY Graph 2"() -> (w1626:cluster{dbl[], dbl[]}[])
            n762 = local read "Slide 2"() -> (w1621:dbl)
            n763 = Decimate 1D Array(w1626) -> (w1623:cluster{dbl[], dbl[]}[], w1622:cluster{dbl[], dbl[]}[])
            n764 = local read "NumPts 2"() -> (w1627:dbl)
            n765 = Array To Cluster(array=w1623) -> (cluster=w1631:T8)
            n766 = Unbundle(w1631) -> ("[0]"=w1630:cluster{dbl[], dbl[]})  [unwired: 8 out]
            n767 = Unbundle(w1630) -> (w1629:dbl[], w1628:dbl[])
            n768 = Array Subset(array=w1629, index=w1621, length=w1627) -> (w1619:dbl[])
            n769 = Array Subset(array=w1628, index=w1621, length=w1627) -> (w1618:dbl[])
            n770 = local write "Index 2"(w1621) -> ()
            n771 = Bundle(w1619, w1618) -> (w1625:cluster{dbl[], dbl[]})  [unwired: 1 in]
            n772 = Build Array (concatenate)(w1623, w1622, w1625) -> (w1624:cluster{dbl[], dbl[]}[])
            n773 = local write "XY Graph 2"(w1624) -> ()
            n774 = local write "Array 7"(w1618) -> ()
            n775 = local write "Array 8"(w1619) -> ()
            n776 = call "sts_calc_subvi.vi"("Array 2"=w1619, "Array"=w1618) -> ("STS"=w1620:dbl)  [unwired: 9 in]
            n777 = local write "New: STS"(w1620) -> ()
          }
          event "Save Changes?": Mouse Down {
            n778 = event-data() -> ()  [unwired: 1 in, 5 out]
            n779 = flat-sequence {
              tunnel: [w1662] -> w1637
              tunnel: [w1661] -> w1635
              tunnel: [w1661] -> w1634
              tunnel: [w1644] -> w1632
              tunnel: w1637 -> [w1776]
              tunnel: [w1777] -> w1636
              tunnel: w1635 -> [w1777]
              tunnel: w1634 -> [w1775]
              tunnel: [w1773] -> w1633
              tunnel: w1632 -> [w1773]
              tunnel: w1636 -> [w1782]
              tunnel: w1633 -> [w1781]
              frame #0 {
                w1649 = -1
                w1642 = "S.T.S. (V/decade):"
                w1643 = "Threshold V (V):"
                (unwired) 3
                w1647 = 1
                n780 = local read "New: Mobility-Sat"() -> (w1684:dbl)
                n781 = local read "Data File"() -> (w1662:path)
                n782 = local read "New: Width"() -> (w1675:dbl)
                n783 = local read "New: Dielectric"() -> (w1685:dbl)
                n784 = local read "New: Length"() -> (w1673:dbl)
                n785 = flat-sequence {
                  tunnel: [w1704] -> w1641
                  tunnel: w1641 -> [w1721]
                  frame #0 {
                    # "Makes Empty File for Transformer Data"
                    n786 = local read "Data Folder"() -> (w1693:path)
                    n787 = Build Path(base path=w1693, name or relative path="Stats") -> (appended path=w1695:path)
                    n788 = call <vilib>:"Check if File or Folder Exists.vi"("path"=w1695) -> ("file or folder exists?"=w1696:bool, "dup path"=w1697:path)  [unwired: 8 in, 1 out]
                    n789 = case shown="False" w1696 {
                      tunnel: [w1701 w1703] -> w1698
                      tunnel: w1697 -> [w1702 w1703]
                      frame False {
                        n790 = Create Folder(path (use dialog)=w1702) -> (created path=w1701:path)  [unwired: 2 in, 2 out]
                      }
                      frame True {
                      }
                    }
                    n791 = Build Path(base path=w1698, name or relative path="Tranformer Data.txt") -> (appended path=w1700:path)
                    n792 = call-poly <vilib>:"Write To Spreadsheet File.vi"("append to file? (new file:F)"=TRUE, "file path (dialog if empty)"=w1700) -> ()  [unwired: 6 in, 1 out]
                  }
                  frame #1 {
                    # "Adds Headers if they don't exist"
                    n793 = Concatenate Strings("Stats\\", "Tranformer Data.txt") -> (w1711:string)
                    n794 = local read "Data Folder"() -> (w1710:path)
                    n795 = Build Path(base path=w1710, name or relative path=w1711) -> (appended path=w1704:path)
                    n796 = call-poly <vilib>:"Read From Spreadsheet File.vi"("file path (dialog if empty)"=w1704) -> ("first row"=w1709:string[])  [unwired: 6 in, 4 out]
                    n797 = Search 1D Array(1D array=w1709, element="DeviceID") -> (index of element=w1707:i32)  [unwired: 1 in]
                    n798 = Equal?(x=w1707, y=0) -> (x = y?=w1705:bool)
                    n799 = case shown="False" w1705 {
                      tunnel: w1704 -> [w1715 _]
                      frame False {
                        n800 = local read "Transformer \nHeaders"() -> (w1714:string[])
                        n801 = call-poly <vilib>:"Write To Spreadsheet File.vi"("1D data"=w1714, "file path (dialog if empty)"=w1715) -> ()  [unwired: 6 in, 1 out]
                      }
                      frame True {
                      }
                    }
                  }
                  frame #2 {
                    # "Adds current device if it doesn't exist"
                    n802 = local read "Current \nRecord"() -> (w1720:string[])
                    n803 = Index Array(array=w1720, index=0) -> (element=w1719:string)
                    n804 = Concatenate Strings("Stats\\", "Tranformer Data.txt") -> (w1724:string)
                    n805 = local read "Data Folder"() -> (w1723:path)
                    n806 = local write "Current Device ID"(w1719) -> ()
                    n807 = local read "Current Device ID"() -> (w1729:string)
                    n808 = Build Path(base path=w1723, name or relative path=w1724) -> (appended path=w1722:path)
                    n809 = call-poly <vilib>:"Read From Spreadsheet File.vi"("file path (dialog if empty)"=w1722) -> ("all rows"=w1716:string[][])  [unwired: 6 in, 4 out]
                    n810 = Index Array(array=w1716, index (col)=0) -> (element=w1717:string[])  [unwired: 1 in]
                    n811 = Search 1D Array(1D array=w1717, element=w1729) -> (index of element=w1718:i32)  [unwired: 1 in]
                    n812 = Equal?(x=w1718, y=-1) -> (x = y?=w1731:bool)
                    n813 = case shown="False" w1731 {
                      tunnel: w1721 -> [w1734 w1745]
                      tunnel: w1718 -> [w1737 _]
                      tunnel: w1716 -> [w1738 _]
                      frame False {
                        n814 = local read "Current \nRecord"() -> (w1736:string[])
                        n815 = Replace Array Subset(array=w1738, new element=w1736, index (row)=w1737) -> (w1735:string[][])  [unwired: 1 in]
                        n816 = flat-sequence {
                          tunnel: w1734 -> [w1739]
                          tunnel: w1735 -> [w1740]
                          tunnel: [w1740] -> w1733
                          tunnel: [w1739] -> w1732
                          tunnel: w1733 -> [w1742]
                          tunnel: w1732 -> [w1741]
                          frame #0 {
                            n817 = Delete(path (use dialog)=w1739) -> ()  [unwired: 4 in, 3 out]
                          }
                          frame #1 {
                            n818 = call-poly <vilib>:"Write To Spreadsheet File.vi"("append to file? (new file:F)"=TRUE, "2D data"=w1742, "file path (dialog if empty)"=w1741) -> ()  [unwired: 5 in, 1 out]
                          }
                        }
                      }
                      frame True {
                        n819 = local read "Current \nRecord"() -> (w1744:string[])
                        n820 = call-poly <vilib>:"Write To Spreadsheet File.vi"("append to file? (new file:F)"=TRUE, "1D data"=w1744, "file path (dialog if empty)"=w1745) -> ()  [unwired: 5 in, 1 out]
                      }
                    }
                  }
                }
                n821 = call-poly <vilib>:"Read From Spreadsheet File.vi"("file path (dialog if empty)"=w1662) -> ("all rows"=w1654:string[][])  [unwired: 6 in, 4 out]
                n822 = Number To Fractional String(number=w1673) -> (F-format string=w1665:string)  [unwired: 3 in]
                n823 = Replace Array Subset(array=w1654, new element=w1665, index (row)=12, index (col)=w1647) -> (w1669:string[][])
                n824 = Number To Fractional String(number=w1675) -> (F-format string=w1676:string)  [unwired: 3 in]
                n825 = Replace Array Subset(array=w1669, new element=w1676, index (row)=13, index (col)=w1647) -> (w1671:string[][])
                n826 = Number To Fractional String(number=w1684) -> (F-format string=w1663:string)  [unwired: 3 in]
                n827 = Number To Fractional String(number=w1685) -> (F-format string=w1664:string)  [unwired: 3 in]
                n828 = Number To Decimal String(number=w1673) -> (decimal integer string=w1672:string)  [unwired: 1 in]
                n829 = local read "Rec: Temp"() -> (w1640:dbl)
                n830 = Equal To 0?(x=w1640) -> (x = 0?=w1639:bool)
                n831 = case shown="False" w1639 {
                  tunnel: [w1688 ""] -> w1638
                  frame False {
                    n832 = local read "Rec: Temp"() -> (w1690:dbl)
                    n833 = Number To Decimal String(number=w1690) -> (decimal integer string=w1687:string)  [unwired: 1 in]
                    n834 = Concatenate Strings("_", w1687, "K") -> (w1688:string)
                  }
                  frame True {
                  }
                }
                n835 = Strip Path(path=w1662) -> (stripped path=w1683:path)  [unwired: 1 out]
                n836 = local read "Index"() -> (w1678:string)
                n837 = Replace Array Subset(array=w1671, new element=w1663, index (row)=15, index (col)=w1647) -> (w1670:string[][])
                n838 = Number To Decimal String(number=w1675) -> (decimal integer string=w1674:string)  [unwired: 1 in]
                n839 = Path To String(path=w1683) -> (string=w1681:string)
                n840 = Replace Array Subset(array=w1670, new element=w1664, index (row)=7, index (col)=w1647) -> (w1646:string[][])
                n841 = call "Build Text"("Temp"=w1638, "Index"=w1678, "Length"=w1672, "Width"=w1674) -> ("Result"=w1679:string)  [unwired: 10 in, 1 out]
                n842 = Concatenate Strings(w1681, "\\", w1679) -> (w1680:string)
                n843 = String To Path(string=w1680) -> (path=w1661:path)
                n844 = Array Size(array=w1654) -> (size(s)=w1656:i32[])
                n845 = Index Array(array=w1656, index=0) -> (element=w1655:i32)
                n846 = Array Subset(array=w1654, index (row)=0, index (col)=0) -> (w1660:string[][])  [unwired: 2 in]
                n847 = Reshape Array(w1660, w1655) -> (w1648:string[])
                n848 = Search 1D Array(1D array=w1648, element=w1643) -> (index of element=w1652:i32)  [unwired: 1 in]
                n849 = Search 1D Array(1D array=w1648, element=w1642) -> (index of element=w1653:i32)  [unwired: 1 in]
                n850 = Equal?(x=w1652, y=w1649) -> (x = y?=w1650:bool)
                n851 = Equal?(x=w1653, y=w1649) -> (x = y?=w1651:bool)
                n852 = case shown="True" w1650 {
                  tunnel: w1652 -> [_ _]
                  tunnel: w1646 -> [w1763 w1771]
                  tunnel: [w1762 w1770] -> w1645
                  tunnel: w1643 -> [_ w1769]
                  frame False {
                    n853 = local read "New: VT"() -> (w1765:dbl)
                    n854 = Number To Fractional String(number=w1765) -> (F-format string=w1761:string)  [unwired: 3 in]
                    n855 = Replace Array Subset(array=w1763, new element=w1761, index (row)=17, index (col)=1) -> (w1762:string[][])
                  }
                  frame True {
                    n856 = local read "New: VT"() -> (w1772:dbl)
                    n857 = Number To Fractional String(number=w1772) -> (F-format string=w1768:string)  [unwired: 3 in]
                    n858 = Build Array(w1769, w1768) -> (w1767:string[])
                    n859 = Insert Into Array(array=w1771, index (row)=17, new element=w1767) -> (w1770:string[][])  [unwired: 1 in]
                  }
                }
                n860 = case shown="True" w1651 {
                  tunnel: w1653 -> [_ _]
                  tunnel: w1645 -> [w1750 w1758]
                  tunnel: [w1749 w1757] -> w1644
                  tunnel: w1642 -> [_ w1755]
                  frame False {
                    n861 = local read "New: STS"() -> (w1752:dbl)
                    n862 = Number To Fractional String(number=w1752) -> (F-format string=w1748:string)  [unwired: 3 in]
                    n863 = Replace Array Subset(array=w1750, new element=w1748, index (row)=18, index (col)=1) -> (w1749:string[][])
                  }
                  frame True {
                    n864 = local read "New: STS"() -> (w1759:dbl)
                    n865 = Number To Fractional String(number=w1759) -> (F-format string=w1756:string)  [unwired: 3 in]
                    n866 = Build Array(w1755, w1756) -> (w1754:string[])
                    n867 = Insert Into Array(array=w1758, index (row)=18, new element=w1754) -> (w1757:string[][])  [unwired: 1 in]
                  }
                }
              }
              frame #1 {
                n868 = Equal?(x=w1776, y=w1775) -> (x = y?=w1774:bool)
                n869 = case shown="False" w1774 {
                  tunnel: w1776 -> [w1780 _]
                  tunnel: w1775 -> [w1779 _]
                  frame False {
                    n870 = Move(source path=w1780, 9:TRUE, 10:w1779) -> ()  [unwired: 2 in, 3 out]
                  }
                  frame True {
                  }
                }
              }
              frame #2 {
                n871 = local write "Data File"(w1782) -> ()
                n872 = call-poly <vilib>:"Write To Spreadsheet File.vi"("2D data"=w1781, "file path (dialog if empty)"=w1782) -> ()  [unwired: 6 in, 1 out]
              }
            }
          }
          event "Save Changes? 2": Mouse Down {
            n873 = event-data() -> ()  [unwired: 1 in, 5 out]
            n874 = local read "Data File"() -> (w1807:path)
            n875 = call "Recorded Values.vi"("Path"=w1807) -> ("Recorded Char"=w1805:T5, "Recorded Prop"=w1804:T6, "Fabrication Prop"=w1806:T7)  [unwired: 8 in]
            n876 = Unbundle By Name(w1805) -> ("Mobility-Sat"=w1791:dbl, "Moblitity-Lin"=w1790:dbl, "On/Off"=w1789:dbl, "Threshold Voltage"=w1788:dbl, "Onset Voltage"=w1787:dbl, "STS"=w1786:dbl, "Trap Density-VT"=w1785:dbl, "Trap Density-STS"=w1784:dbl)
            n877 = Unbundle By Name(w1806) -> ("Date Created"=w1783:string, "Material"=w1803:string, "Solvent"=w1802:string, "Concentration"=w1801:dbl, "Method"=w1800:string, "Dielectric (nm)"=w1799:dbl, "Treatment"=w1798:string, "Comments"=w1797:string)
            n878 = Unbundle By Name(w1804) -> ("Date Recorded"=w1796:string, "Index"=w1795:string, "Length"=w1794:dbl, "Width"=w1793:dbl, "Sample Temp"=w1792:dbl)
            n879 = local write "Rec: Material"(w1803) -> ()
            n880 = local write "Date Created"(w1783) -> ()
            n881 = local write "Rec: Solvent"(w1802) -> ()
            n882 = local write "Rec: Concentration"(w1801) -> ()
            n883 = local write "Rec: Method"(w1800) -> ()
            n884 = local write "Rec: Dielectric (d)"(w1799) -> ()
            n885 = local write "Surface Treatment:"(w1798) -> ()
            n886 = local write "Comments"(w1797) -> ()
            n887 = local write "Index"(w1795) -> ()
            n888 = local write "Rec: Mobility-Sat"(w1791) -> ()
            n889 = local write "Rec: Mobility-Lin"(w1790) -> ()
            n890 = local write "Rec: On/Off"(w1789) -> ()
            n891 = local write "Rec: VT"(w1788) -> ()
            n892 = local write "Rec: Onset V"(w1787) -> ()
            n893 = local write "Rec: STS"(w1786) -> ()
            n894 = local write "Rec: Trap Density-VT"(w1785) -> ()
            n895 = local write "Rec: Trap Density-STS"(w1784) -> ()
            n896 = stacked-sequence {
              seq-local: [w1887 _ _ _ _] -> [_ w1946 _ _ _]
              seq-local: [w1886 _ _ _ _] -> [_ w1947 _ _ _]
              seq-local: [w1886 _ _ _ _] -> [_ w1945 _ _ _]
              seq-local: [w1869 _ _ _ _] -> [_ w1943 _ _ _]
              seq-local: [_ w1947 _ _ _] -> [_ _ w1952 _ _]
              seq-local: [_ w1943 _ _ _] -> [_ _ w1951 _ _]
              frame #0 {
                w1874 = -1
                w1867 = "STS (V/decade):"
                w1868 = "Threshold V (V):"
                (unwired) 3
                w1872 = 1
                n897 = local read "Data File"() -> (w1887:path)
                n898 = local read "New: Width"() -> (w1900:dbl)
                n899 = local read "New: Dielectric"() -> (w1910:dbl)
                n900 = local read "New: Length"() -> (w1898:dbl)
                n901 = local read "New: Mobility-Sat"() -> (w1909:dbl)
                n902 = local read "Rec: Temp"() -> (w1866:dbl)
                n903 = call-poly <vilib>:"Read From Spreadsheet File.vi"("file path (dialog if empty)"=w1887) -> ("all rows"=w1879:string[][])  [unwired: 6 in, 4 out]
                n904 = Number To Fractional String(number=w1898) -> (F-format string=w1890:string)  [unwired: 3 in]
                n905 = Replace Array Subset(array=w1879, new element=w1890, index (row)=12, index (col)=w1872) -> (w1894:string[][])
                n906 = Number To Fractional String(number=w1909) -> (F-format string=w1888:string)  [unwired: 3 in]
                n907 = Equal To 0?(x=w1866) -> (x = 0?=w1865:bool)
                n908 = Number To Fractional String(number=w1910) -> (F-format string=w1889:string)  [unwired: 3 in]
                n909 = Number To Fractional String(number=w1900) -> (F-format string=w1901:string)  [unwired: 3 in]
                n910 = Replace Array Subset(array=w1894, new element=w1901, index (row)=13, index (col)=w1872) -> (w1896:string[][])
                n911 = Number To Decimal String(number=w1898) -> (decimal integer string=w1897:string)  [unwired: 1 in]
                n912 = case shown="False" w1865 {
                  tunnel: [w1912 ""] -> w1864
                  frame False {
                    n913 = local read "Rec: Temp"() -> (w1915:dbl)
                    n914 = Number To Decimal String(number=w1915) -> (decimal integer string=w1914:string)  [unwired: 1 in]
                    n915 = Concatenate Strings("_", w1914, "K") -> (w1912:string)
                  }
                  frame True {
                  }
                }
                n916 = Strip Path(path=w1887) -> (stripped path=w1908:path)  [unwired: 1 out]
                n917 = local read "Index"() -> (w1903:string)
                n918 = Replace Array Subset(array=w1896, new element=w1888, index (row)=15, index (col)=w1872) -> (w1895:string[][])
                n919 = Number To Decimal String(number=w1900) -> (decimal integer string=w1899:string)  [unwired: 1 in]
                n920 = Path To String(path=w1908) -> (string=w1906:string)
                n921 = Replace Array Subset(array=w1895, new element=w1889, index (row)=7, index (col)=w1872) -> (w1871:string[][])
                n922 = call "Build Text2"("Temp"=w1864, "Index"=w1903, "Length"=w1897, "Width"=w1899) -> ("Result"=w1904:string)  [unwired: 10 in, 1 out]
                n923 = Concatenate Strings(w1906, "\\", w1904) -> (w1905:string)
                n924 = String To Path(string=w1905) -> (path=w1886:path)
                n925 = Array Size(array=w1879) -> (size(s)=w1881:i32[])
                n926 = Index Array(array=w1881, index=0) -> (element=w1880:i32)
                n927 = Array Subset(array=w1879, index (row)=0, index (col)=0) -> (w1885:string[][])  [unwired: 2 in]
                n928 = Reshape Array(w1885, w1880) -> (w1873:string[])
                n929 = Search 1D Array(1D array=w1873, element=w1868) -> (index of element=w1877:i32)  [unwired: 1 in]
                n930 = Search 1D Array(1D array=w1873, element=w1867) -> (index of element=w1878:i32)  [unwired: 1 in]
                n931 = Equal?(x=w1877, y=w1874) -> (x = y?=w1875:bool)
                n932 = Equal?(x=w1878, y=w1874) -> (x = y?=w1876:bool)
                n933 = case shown="True" w1875 {
                  tunnel: w1877 -> [_ _]
                  tunnel: w1871 -> [w1933 w1941]
                  tunnel: [w1932 w1940] -> w1870
                  tunnel: w1868 -> [_ w1939]
                  frame False {
                    n934 = local read "New: VT"() -> (w1935:dbl)
                    n935 = Number To Fractional String(number=w1935) -> (F-format string=w1931:string)  [unwired: 3 in]
                    n936 = Replace Array Subset(array=w1933, new element=w1931, index (row)=17, index (col)=1) -> (w1932:string[][])
                  }
                  frame True {
                    n937 = local read "New: VT"() -> (w1942:dbl)
                    n938 = Number To Fractional String(number=w1942) -> (F-format string=w1938:string)  [unwired: 3 in]
                    n939 = Build Array(w1939, w1938) -> (w1937:string[])
                    n940 = Insert Into Array(array=w1941, index (row)=17, new element=w1937) -> (w1940:string[][])  [unwired: 1 in]
                  }
                }
                n941 = case shown="True" w1876 {
                  tunnel: w1878 -> [_ _]
                  tunnel: w1870 -> [w1920 w1928]
                  tunnel: [w1919 w1927] -> w1869
                  tunnel: w1867 -> [_ w1925]
                  frame False {
                    n942 = local read "New: STS"() -> (w1922:dbl)
                    n943 = Number To Fractional String(number=w1922) -> (F-format string=w1918:string)  [unwired: 3 in]
                    n944 = Replace Array Subset(array=w1920, new element=w1918, index (row)=18, index (col)=1) -> (w1919:string[][])
                  }
                  frame True {
                    n945 = local read "New: STS"() -> (w1929:dbl)
                    n946 = Number To Fractional String(number=w1929) -> (F-format string=w1926:string)  [unwired: 3 in]
                    n947 = Build Array(w1925, w1926) -> (w1924:string[])
                    n948 = Insert Into Array(array=w1928, index (row)=18, new element=w1924) -> (w1927:string[][])  [unwired: 1 in]
                  }
                }
              }
              frame #1 {
                n949 = Equal?(x=w1946, y=w1945) -> (x = y?=w1944:bool)
                n950 = case shown="False" w1944 {
                  tunnel: w1946 -> [w1950 _]
                  tunnel: w1945 -> [w1949 _]
                  frame False {
                    n951 = Move(source path=w1950, 9:TRUE, 10:w1949) -> ()  [unwired: 2 in, 3 out]
                  }
                  frame True {
                  }
                }
              }
              frame #2 {
                n952 = local write "Data File"(w1952) -> ()
                n953 = call-poly <vilib>:"Write To Spreadsheet File.vi"("2D data"=w1951, "file path (dialog if empty)"=w1952) -> ()  [unwired: 6 in, 1 out]
              }
              frame #3 {
                w2008 = 0
                # "Moves to next file and displays new image/data"
                n954 = local read "Data File"() -> (w2013:path)
                n955 = local read "Image Folder"() -> (w1998:path)
                n956 = Strip Path(path=w2013) -> (stripped path=w2004:path, name=w2025:string)
                n957 = local write "Data Folder"(w2004) -> ()
                n958 = List Folder(path=w2004) -> (filenames=w2018:string[])  [unwired: 3 in, 3 out]
                n959 = List Folder(path=w1998) -> (filenames=w2003:string[])  [unwired: 3 in, 3 out]
                n960 = Search 1D Array(1D array=w2018, element=w2025) -> (index of element=w2015:i32)  [unwired: 1 in]
                n961 = Array Size(array=w2018) -> (size(s)=w2014:i32)
                n962 = Decrement(x=w2014) -> (x-1=w2016:i32)
                n963 = local read "Folder Index"() -> (w1954:dbl)
                n964 = Equal?(x=w2015, y=w2016) -> (x = y?=w2017:bool)
                n965 = case shown="False" w2017 {
                  tunnel: w1954 -> [w2148 _]
                  tunnel: [w2147 0] -> w1953
                  frame False {
                    n966 = Increment(x=w2148) -> (x+1=w2147:dbl)
                  }
                  frame True {
                  }
                }
                n967 = property on="Image Out" class="ImageControl"() -> (error out=w1958:errorcluster, "Image Center Position"=w1962:cluster{"X":u32, "Y":u32})  [unwired: 2 in, 1 out]
                n968 = Path To String(path=w2004) -> (string=w2026:string)
                n969 = Index Array(array=w2018, index=w1953) -> (element=w2019:string)
                n970 = local write "Folder Index"(w1953) -> ()
                n971 = local write "Data Name:"(w2019) -> ()
                n972 = Unbundle(w1962) -> ("X"=w1960:u32)  [unwired: 1 out]
                n973 = Concatenate Strings(w2026, "\\", w2019) -> (w2024:string)
                n974 = Bundle("X"=w1960, 0) -> (w1961:cluster{"X":u32, i32})  [unwired: 1 in]
                n975 = String To Path(string=w2024) -> (path=w1980:path)
                n976 = property on="Image Out" class="ImageControl"(error in=w1958, "Image Center Position"=w1961) -> ()  [unwired: 1 in, 2 out]
                n977 = local read "NumPts 2"() -> (w1973:dbl)
                n978 = local write "Data File"(w1980) -> ()
                n979 = local read "NumPts"() -> (w1979:dbl)
                n980 = call-poly <vilib>:"Read From Spreadsheet File.vi"("file path (dialog if empty)"=w1980) -> ("all rows"=w2010:string[][])  [unwired: 6 in, 4 out]
                n981 = call "sub_thresh_swing_subvi.vi"("Path"=w1980, "NumPts"=w1973) -> ("Index"=w1974:dbl, "XY Graph"=w1969:cluster{dbl[], dbl[]}[], "Sub Threshold Swing"=w1981:dbl)  [unwired: 9 in, 2 out]
                n982 = call "mobility_subvi_07_12a_JW.vi"("Path"=w1980, "NumPts"=w1979) -> ("Dielectric (d)"=w1984:dbl, "Index"=w1989:dbl, "XY Graph"=w1992:cluster{dbl[], dbl[]}[], "Length"=w1982:dbl, "Vt"=w1985:dbl, "Width"=w1983:dbl, "Table Control"=w2022:string[][], "Table Control 2"=w2021:string[][], "Mobility"=w2020:dbl)  [unwired: 4 in, 1 out]
                n983 = local write "Index 2"(w1974) -> ()
                n984 = local write "Calc: STS"(w1981) -> ()
                n985 = local write "XY Graph"(w1992) -> ()
                n986 = local write "Slide"(w1989) -> ()
                n987 = local write "Calc: VT"(w1985) -> ()
                n988 = Array Size(array=w2010) -> (size(s)=w2009:i32[])
                n989 = local write "XY Graph 2"(w1969) -> ()
                n990 = Decimate 1D Array(w1969) -> (w1972:cluster{dbl[], dbl[]}[])  [unwired: 1 out]
                n991 = Decimate 1D Array(w1992) -> (w1993:cluster{dbl[], dbl[]}[])  [unwired: 1 out]
                n992 = local write "New: Length"(w1982) -> ()
                n993 = local write "MobVi Index"(w1989) -> ()
                n994 = local write "New: Dielectric"(w1984) -> ()
                n995 = local write "Table Control 2"(w2021) -> ()
                n996 = Index Array(array=w2009, index=w2008) -> (element=w1987:i32)
                n997 = Array Subset(array=w2010, index (row)=w2008, index (col)=w2008, length (col)=3) -> (w2011:string[][])  [unwired: 1 in]
                n998 = local write "New: Width"(w1983) -> ()
                n999 = local write "Calc: Mobility-Sat"(w2020) -> ()
                n1000 = local write "Table Control"(w2022) -> ()
                n1001 = Array To Cluster(array=w1972) -> (cluster=w1970:T8)
                n1002 = Array To Cluster(array=w1993) -> (cluster=w1995:T8)
                n1003 = Reshape Array(w2011, w1987) -> (w1996:string[])
                n1004 = Subtract(x=w1987, y=20) -> (x-y=w1986:i32)
                n1005 = property on="Slide" class="Slide (strict)"("Scale.Maximum"=w1986) -> ()  [unwired: 2 in, 2 out]
                n1006 = Unbundle(w1970) -> ("[0]"=w1971:cluster{dbl[], dbl[]})  [unwired: 8 out]
                n1007 = Unbundle(w1995) -> ("[0]"=w1994:cluster{dbl[], dbl[]})  [unwired: 8 out]
                n1008 = Unbundle(w1971) -> (w1968:dbl[], w1967:dbl[])
                n1009 = Unbundle(w1994) -> (w1976:dbl[], w1975:dbl[])
                n1010 = Array Subset(array=w1968, index=w1974, length=w1973) -> (w1978:dbl[])
                n1011 = Array Subset(array=w1967, index=w1974, length=w1973) -> (w1977:dbl[])
                n1012 = Array Subset(array=w1976, index=w1989, length=w1979) -> (w1991:dbl[])
                n1013 = Array Subset(array=w1975, index=w1989, length=w1979) -> (w1990:dbl[])
                n1014 = local write "Array 8"(w1978) -> ()
                n1015 = local write "Array 7"(w1977) -> ()
                n1016 = local write "Array"(w1991) -> ()
                n1017 = local write "Array 2"(w1990) -> ()
                n1018 = Search 1D Array(1D array=w1996, element="Index:") -> (index of element=w2005:i32)  [unwired: 1 in]
                n1019 = Increment(x=w2005) -> (x+1=w2006:i32)
                n1020 = Index Array(array=w1996, index=w2006) -> (element=w2001:string)
                n1021 = while {
                  tunnel: w2003 -> [w2034]
                  tunnel: w2001 -> [w2032]
                  tunnel: [w2031] -> _
                  tunnel: [w2031] -> w2002
                  tunnel: w1987 -> [w2030]
                  i -> [w2031]
                  stop <- w2027 stop-if-true
                  n1022 = Index Array(array=w2034, index=w2031) -> (element=w2035:string)
                  n1023 = xnode "Match Regular Expression"("input string"=w2035, "regular expression"=w2032) -> ("whole match"=w2033:string)  [unwired: 4 in, 4 out]
                  n1024 = Equal?(x=w2033, y=w2032) -> (x = y?=w2029:bool)
                  n1025 = Equal?(x=w2030, y=w2031) -> (x = y?=w2028:bool)
                  n1026 = Or(x=w2029, y=w2028) -> (x .or. y?=w2027:bool)
                }
                n1027 = local write "Index"(w2001) -> ()
                n1028 = local read "No Image"() -> (w1963:path)
                n1029 = Path To String(path=w1998) -> (string=w2000:string)
                n1030 = local read "Image Out"() -> (w1955:T2)
                n1031 = Index Array(array=w2003, index=w2002) -> (element=w1965:string)
                n1032 = Empty String/Path?(string/path=w1965) -> (empty?=w1966:bool)
                n1033 = Concatenate Strings(w2000, "\\", w1965) -> (w1999:string)
                n1034 = local write "Image Name"(w1965) -> ()
                n1035 = String To Path(string=w1999) -> (path=w1964:path)
                n1036 = Select(t=w1963, s=w1966, f=w1964) -> (s? t:f=w1957:path)
                n1037 = local write "Image File"(w1957) -> ()
                n1038 = call "IMAQ ReadFile"("File Path"=w1957, "Image"=w1955) -> ("Image Out"=w1956:T2)  [unwired: 5 in, 4 out]
                n1039 = local write "Image Out 2"(w1956) -> ()
                n1040 = local write "Image Out"(w1956) -> ()
                n1041 = invoke on="Image Out" class="ImageControl" method="Clear ROI"() -> ()  [unwired: 3 in, 3 out]
              }
              frame #4 {
                # "Output ROI data"
                n1042 = local read "Image Folder"() -> (w2150:path)
                n1043 = Build Path(base path=w2150, name or relative path="ROI") -> (appended path=w2152:path)
                n1044 = local read "Index"() -> (w2151:string)
                n1045 = Build Path(base path=w2152, name or relative path=w2151) -> (appended path=w2157:path)
                n1046 = invoke on="Image Out" class="ImageControl" method="Clear ROI"() -> (error out=w2156:errorcluster)  [unwired: 3 in, 2 out]
                n1047 = call <vilib>:"Check if File or Folder Exists.vi"("error in (no error)"=w2156, "path"=w2157) -> ("file or folder exists?"=w2154:bool, "dup path"=w2155:path)  [unwired: 7 in, 1 out]
                n1048 = case shown="True" w2154 {
                  tunnel: w2155 -> [_ w2158]
                  frame False {
                  }
                  frame True {
                    n1049 = Read from Text File(file (use dialog)=w2158) -> (text=w2162:string)  [unwired: 3 in, 3 out]
                    n1050 = property on="Image Out" class="ImageControl"() -> ("ROI"=w2159:T9)  [unwired: 2 in, 2 out]
                    n1051 = Unflatten From String(type=w2159, binary string=w2162) -> (value=w2160:T9, error out=w2161:errorcluster)  [unwired: 3 in, 1 out]
                    n1052 = property on="Image Out" class="ImageControl"(error in=w2161, "ROI"=w2160) -> ()  [unwired: 1 in, 2 out]
                  }
                }
              }
            }
            n1053 = local write "Date Recorded"(w1796) -> ()
            n1054 = local write "Rec: Length"(w1794) -> ()
            n1055 = local write "Rec: Width"(w1793) -> ()
            n1056 = local write "Rec: Temp"(w1792) -> ()
            n1057 = flat-sequence {
              tunnel: [w1821] -> w1808
              tunnel: w1808 -> [w1835]
              frame #0 {
                # "Makes Empty File for Transformer Data"
                n1058 = local read "Data Folder"() -> (w1810:path)
                n1059 = Build Path(base path=w1810, name or relative path="Stats") -> (appended path=w1812:path)
                n1060 = call <vilib>:"Check if File or Folder Exists.vi"("path"=w1812) -> ("file or folder exists?"=w1813:bool, "dup path"=w1814:path)  [unwired: 8 in, 1 out]
                n1061 = case shown="False" w1813 {
                  tunnel: [w1818 w1820] -> w1815
                  tunnel: w1814 -> [w1819 w1820]
                  frame False {
                    n1062 = Create Folder(path (use dialog)=w1819) -> (created path=w1818:path)  [unwired: 2 in, 2 out]
                  }
                  frame True {
                  }
                }
                n1063 = Build Path(base path=w1815, name or relative path="Tranformer Data.txt") -> (appended path=w1817:path)
                n1064 = call-poly <vilib>:"Write To Spreadsheet File.vi"("append to file? (new file:F)"=TRUE, "file path (dialog if empty)"=w1817) -> ()  [unwired: 6 in, 1 out]
              }
              frame #1 {
                # "Adds Headers if they don't exist"
                n1065 = Concatenate Strings("Stats\\", "Tranformer Data.txt") -> (w1828:string)
                n1066 = local read "Data Folder"() -> (w1827:path)
                n1067 = Build Path(base path=w1827, name or relative path=w1828) -> (appended path=w1821:path)
                n1068 = call-poly <vilib>:"Read From Spreadsheet File.vi"("file path (dialog if empty)"=w1821) -> ("first row"=w1826:string[])  [unwired: 6 in, 4 out]
                n1069 = Search 1D Array(1D array=w1826, element="DeviceID") -> (index of element=w1824:i32)  [unwired: 1 in]
                n1070 = Equal?(x=w1824, y=0) -> (x = y?=w1822:bool)
                n1071 = case shown="False" w1822 {
                  tunnel: w1821 -> [w1832 _]
                  frame False {
                    n1072 = local read "Transformer \nHeaders"() -> (w1831:string[])
                    n1073 = call-poly <vilib>:"Write To Spreadsheet File.vi"("1D data"=w1831, "file path (dialog if empty)"=w1832) -> ()  [unwired: 6 in, 1 out]
                  }
                  frame True {
                  }
                }
              }
              frame #2 {
                # "Adds current device if it doesn't exist"
                n1074 = local read "Current \nRecord"() -> (w1838:string[])
                n1075 = Index Array(array=w1838, index=0) -> (element=w1837:string)
                n1076 = Concatenate Strings("Stats\\", "Tranformer Data.txt") -> (w1841:string)
                n1077 = local read "Data Folder"() -> (w1840:path)
                n1078 = local write "Current Device ID"(w1837) -> ()
                n1079 = local read "Current Device ID"() -> (w1847:string)
                n1080 = Build Path(base path=w1840, name or relative path=w1841) -> (appended path=w1839:path)
                n1081 = call-poly <vilib>:"Read From Spreadsheet File.vi"("file path (dialog if empty)"=w1839) -> ("all rows"=w1834:string[][])  [unwired: 6 in, 4 out]
                n1082 = Index Array(array=w1834, index (col)=0) -> (element=w1845:string[])  [unwired: 1 in]
                n1083 = Search 1D Array(1D array=w1845, element=w1847) -> (index of element=w1833:i32)  [unwired: 1 in]
                n1084 = Equal?(x=w1833, y=-1) -> (x = y?=w1836:bool)
                n1085 = case shown="False" w1836 {
                  tunnel: w1835 -> [w1849 w1862]
                  tunnel: w1833 -> [w1854 _]
                  tunnel: w1834 -> [w1855 _]
                  frame False {
                    n1086 = local read "Current \nRecord"() -> (w1853:string[])
                    n1087 = Replace Array Subset(array=w1855, new element=w1853, index (row)=w1854) -> (w1850:string[][])  [unwired: 1 in]
                    n1088 = flat-sequence {
                      tunnel: [w1856] -> _
                      tunnel: [w1857] -> _
                      tunnel: [w1857] -> w1852
                      tunnel: [w1856] -> w1851
                      tunnel: w1850 -> [w1857]
                      tunnel: w1849 -> [w1856]
                      tunnel: w1852 -> [w1859]
                      tunnel: w1851 -> [w1858]
                      frame #0 {
                        n1089 = Delete(path (use dialog)=w1856) -> ()  [unwired: 4 in, 3 out]
                      }
                      frame #1 {
                        n1090 = call-poly <vilib>:"Write To Spreadsheet File.vi"("append to file? (new file:F)"=TRUE, "2D data"=w1859, "file path (dialog if empty)"=w1858) -> ()  [unwired: 5 in, 1 out]
                      }
                    }
                  }
                  frame True {
                    n1091 = local read "Current \nRecord"() -> (w1861:string[])
                    n1092 = call-poly <vilib>:"Write To Spreadsheet File.vi"("append to file? (new file:F)"=TRUE, "1D data"=w1861, "file path (dialog if empty)"=w1862) -> ()  [unwired: 5 in, 1 out]
                  }
                }
              }
            }
          }
          event "Export": Mouse Down {
            n1093 = event-data() -> ()  [unwired: 1 in, 7 out]
            n1094 = call "OA_ConnectToOrigin.vi"() -> ("error out"=w2184:errorcluster, "Origin.IOApplication"=w2185:refnum<k7>)  [unwired: 8 in]
            n1095 = local read "Data Folder"() -> (w2163:path)
            n1096 = local read "Project"() -> (w2183:path)
            n1097 = call "OA_Load.vi"("error in (no error)"=w2184, "Path"=w2183, "Origin.IOApplication"=w2185) -> ("error out"=w2176:errorcluster, "Origin.IOApplication"=w2177:refnum<k7>)  [unwired: 1 out]
            n1098 = call "OAExecute.vi"("script"="document -m 3;", "Error IO"=w2176, "Origin.IOApplication"=w2177) -> ("Error IO Out"=w2174:errorcluster, "Origin.IOApplication"=w2175:refnum<k7>)  [unwired: 1 in, 1 out]
            n1099 = Build Path(base path=w2163, name or relative path="Stats") -> (appended path=w2164:path)
            n1100 = call <vilib>:"Check if File or Folder Exists.vi"("path"=w2164) -> ("file or folder exists?"=w2189:bool, "dup path"=w2188:path)  [unwired: 8 in, 1 out]
            n1101 = case shown="False" w2189 {
              tunnel: w2188 -> [w2249 w2250]
              tunnel: [w2248 w2250] -> w2182
              frame False {
                n1102 = Create Folder(path (use dialog)=w2249) -> (created path=w2248:path)  [unwired: 2 in, 2 out]
              }
              frame True {
              }
            }
            n1103 = flat-sequence {
              tunnel: w2163 -> [w2205]
              tunnel: w2182 -> [w2204]
              tunnel: [w2194] -> w2187
              tunnel: [w2195] -> w2186
              tunnel: w2175 -> [w2199]
              tunnel: w2174 -> [w2198]
              tunnel: w2163 -> [w2221]
              tunnel: w2182 -> [w2220]
              tunnel: w2187 -> [w2216]
              tunnel: w2186 -> [w2217]
              tunnel: [w2211] -> w2181
              tunnel: [w2210] -> w2180
              tunnel: w2163 -> [w2232]
              tunnel: w2182 -> [w2231]
              tunnel: w2181 -> [w2227]
              tunnel: w2180 -> [w2226]
              tunnel: [w2225] -> w2179
              tunnel: [w2224] -> w2178
              tunnel: w2163 -> [w2247]
              tunnel: w2182 -> [w2246]
              tunnel: w2179 -> [w2241]
              tunnel: w2178 -> [w2240]
              tunnel: [w2238] -> w2172
              tunnel: [w2237] -> w2171
              frame #0 {
                n1104 = call "Param_Analysis.vi"("error in (no error)"=w2198, "Folder 2"=w2205, "Parameter String"="Mobility (cm^2/Vs):", "Parameter Name"="Mobility", "Folder"=w2204) -> ("error out"=w2201:errorcluster, "Array 4"=w2191:string[], "Array 3"=w2200:string[][])  [unwired: 3 in, 1 out]
                n1105 = call "Origin_Export.vi"("String 3"="[MobHistTab]Sheet1", "error in (no error)"=w2201, "Array"=w2200, "String 2"="[MOBvsLTable]Mobilities", "String"="pe_cd \"Mobility Chart\";", "Origin.IOApplication"=w2199, "Array 2"=w2191) -> ("reference out"=w2197:refnum<k7>, "error out"=w2196:errorcluster)  [unwired: 2 in, 1 out]
                n1106 = call "OAExecute.vi"("script"="window -a MOBvsLTable;\nwindow -s TV;", "Error IO"=w2196, "Origin.IOApplication"=w2197) -> ("Error IO Out"=w2194:errorcluster, "Origin.IOApplication"=w2195:refnum<k7>)  [unwired: 1 in, 1 out]
              }
              frame #1 {
                n1107 = call "Param_Analysis.vi"("error in (no error)"=w2216, "Folder 2"=w2221, "Parameter String"="On/Off Current:", "Parameter Name"="On_Off_Current", "Folder"=w2220) -> ("error out"=w2215:errorcluster, "Array 4"=w2209:string[], "Array 3"=w2212:string[][])  [unwired: 3 in, 1 out]
                n1108 = call "Origin_Export.vi"("String 3"="[OnOffHistTab]Sheet1", "error in (no error)"=w2215, "Array"=w2212, "String 2"="[OnOffTable]On/Off Ratios", "String"="pe_cd \"OnOff vs L\";", "Origin.IOApplication"=w2217, "Array 2"=w2209) -> ("reference out"=w2211:refnum<k7>, "error out"=w2210:errorcluster)  [unwired: 2 in, 1 out]
              }
              frame #2 {
                n1109 = call "Param_Analysis.vi"("Folder 2"=w2232, "Parameter String"="S.T.S. (V/decade):", "Parameter Name"="STS", "Folder"=w2231) -> ("Array 4"=w2223:string[], "Array 3"=w2228:string[][])  [unwired: 4 in, 2 out]
                n1110 = call "Origin_Export.vi"("String 3"="[SHistTab]Sheet1", "error in (no error)"=w2226, "Array"=w2228, "String 2"="[STable]Threshold Swing", "String"="pe_cd \"Threshold Swing vs L\";", "Origin.IOApplication"=w2227, "Array 2"=w2223) -> ("reference out"=w2224:refnum<k7>, "error out"=w2225:errorcluster)  [unwired: 2 in, 1 out]
              }
              frame #3 {
                n1111 = call "Param_Analysis.vi"("Folder 2"=w2247, "Parameter String"="Threshold V (V):", "Parameter Name"="Threshold_V", "Folder"=w2246) -> ("Array 4"=w2236:string[], "Array 3"=w2239:string[][])  [unwired: 4 in, 2 out]
                n1112 = call "Origin_Export.vi"("String 3"="[VtHistTab]Sheet1", "error in (no error)"=w2241, "Array"=w2239, "String 2"="[VtTable]Threshold Voltages", "String"="pe_cd \"Threshold Voltage vs L\";", "Origin.IOApplication"=w2240, "Array 2"=w2236) -> ("reference out"=w2238:refnum<k7>, "error out"=w2237:errorcluster)  [unwired: 2 in, 1 out]
              }
            }
            n1113 = call "File Dialog"("start path"=w2164) -> ("selected path"=w2167:path)  [unwired: 11 in, 3 out]
            n1114 = Path To String(path=w2167) -> (string=w2166:string)
            n1115 = call "OAExecute.vi"("script"="pe_cd /;\npe_cd \"Mobility Chart\"; ", "Error IO"=w2171, "Origin.IOApplication"=w2172) -> ("Error IO Out"=w2168:errorcluster, "Origin.IOApplication"=w2169:refnum<k7>)  [unwired: 1 in, 1 out]
            n1116 = call "OASaveProject.vi"("path"=w2166, "Error IO"=w2168, "Origin.IOApplication"=w2169) -> ()  [unwired: 3 out]
          }
          event "Blank Button": Mouse Down {
            n1117 = event-data() -> ()  [unwired: 1 in, 7 out]
            n1118 = local read "Data File"() -> (w2258:path)
            n1119 = Strip Path(path=w2258) -> (stripped path=w2254:path, name=w2256:string)
            n1120 = Path To String(path=w2254) -> (string=w2253:string)
            n1121 = Concatenate Strings(w2253, "\\", "X_", w2256) -> (w2252:string)
            n1122 = String To Path(string=w2252) -> (path=w2251:path)
            n1123 = Move(source path=w2258, 10:w2251) -> ()  [unwired: 3 in, 3 out]
            n1124 = local write "Data File"(w2251) -> ()
          }
          event "Cancel Button": Mouse Down {
            (unwired) 6
            n1125 = event-data() -> ()  [unwired: 1 in, 7 out]
            n1126 = call "Simulate_Keyboard.vi"("Action"=2, "Virtual Key"=162) -> ()  [unwired: 7 in, 1 out]
          }
        }
        n1127 = Reciprocal(x=w487) -> (1/x=w486:sgl)
        n1128 = Multiply(x=w486, y=10) -> (x*y=w488:sgl)
        n1129 = case shown="\"EQUALS\"" w527 {
          tunnel: w501 -> [w576 w582 w586 w588 w592 w594 w596 w598 w600 w602 w604 w606 w608 w610 w612 w614 w616 w618 w620 w622 w624 w626 w628 w630 w632 w634 w636 w638 w640 w642 w644 w646 w648 w650 w652 w654 w656 w658 w660 w662 w664 w666 w668 w670 w672 w674 w676 w678 w680 w682 w684 w686 w688 w690 w692 w694 w696 w698 w700 w702 w704 w706 w708 w710 w712 w714 w716 w718 w720 w722 w724 w726 w728 w730 w732 w734 w736 w738 w740 w742 w744 w746 w748 w750 w752 w754 w756 w758 w760 w762 w764 w766 w768 w770 w772 w774 w776 w778 w780 w782 w784 w786 w788 w790 w792]
          tunnel: [w576 w581 w585 w588 w592 w594 w596 w598 w600 w602 w604 w606 w608 w610 w612 w614 w616 w618 w620 w622 w624 w626 w628 w630 w632 w634 w636 w638 w640 w642 w644 w646 w648 w650 w652 w654 w656 w658 w660 w662 w664 w666 w668 w670 w672 w674 w676 w678 w680 w682 w684 w686 w688 w690 w692 w694 w696 w698 w700 w702 w704 w706 w708 w710 w712 w714 w716 w718 w720 w722 w724 w726 w728 w730 w732 w734 w736 w738 w740 w742 w744 w746 w748 w750 w752 w754 w756 w758 w760 w762 w764 w766 w768 w770 w772 w774 w776 w778 w780 w782 w784 w786 w788 w790 w792] -> w526
          tunnel: w502 -> [w578 w580 w584 w590 w591 w593 w595 w597 w599 w601 w603 w605 w607 w609 w611 w613 w615 w617 w619 w621 w623 w625 w627 w629 w631 w633 w635 w637 w639 w641 w643 w645 w647 w649 w651 w653 w655 w657 w659 w661 w663 w665 w667 w669 w671 w673 w675 w677 w679 w681 w683 w685 w687 w689 w691 w693 w695 w697 w699 w701 w703 w705 w707 w709 w711 w713 w715 w717 w719 w721 w723 w725 w727 w729 w731 w733 w735 w737 w739 w741 w743 w745 w747 w749 w751 w753 w755 w757 w759 w761 w763 w765 w767 w769 w771 w773 w775 w777 w779 w781 w783 w785 w787 w789 w791]
          tunnel: [w577 w580 w584 w589 w591 w593 w595 w597 w599 w601 w603 w605 w607 w609 w611 w613 w615 w617 w619 w621 w623 w625 w627 w629 w631 w633 w635 w637 w639 w641 w643 w645 w647 w649 w651 w653 w655 w657 w659 w661 w663 w665 w667 w669 w671 w673 w675 w677 w679 w681 w683 w685 w687 w689 w691 w693 w695 w697 w699 w701 w703 w705 w707 w709 w711 w713 w715 w717 w719 w721 w723 w725 w727 w729 w731 w733 w735 w737 w739 w741 w743 w745 w747 w749 w751 w753 w755 w757 w759 w761 w763 w765 w767 w769 w771 w773 w775 w777 w779 w781 w783 w785 w787 w789 w791] -> w525
          tunnel: w488 -> [w575 w579 w583 w587 _ _ _ _ _ _ _ _ _ _ _ _ _ _ _ _ _ _ _ _ _ _ _ _ _ _ _ _ _ _ _ _ _ _ _ _ _ _ _ _ _ _ _ _ _ _ _ _ _ _ _ _ _ _ _ _ _ _ _ _ _ _ _ _ _ _ _ _ _ _ _ _ _ _ _ _ _ _ _ _ _ _ _ _ _ _ _ _ _ _ _ _ _ _ _ _ _ _ _ _ _]
          frame "DOWN" {
            n1130 = Add(x=w578, y=w575) -> (x+y=w577:sgl)
          }
          frame "LEFT" {
            n1131 = Subtract(x=w582, y=w579) -> (x-y=w581:sgl)
          }
          frame "RIGHT" {
            n1132 = Add(x=w586, y=w583) -> (x+y=w585:sgl)
          }
          frame "UP" {
            n1133 = Subtract(x=w590, y=w587) -> (x-y=w589:sgl)
          }
          frame "ENTER (num pad)" {
          }
          frame "' (quote)" {
          }
          frame "END" {
          }
          frame "EQUALS" {
          }
          frame "ESCAPE" {
          }
          frame "GRAVE (`)" {
          }
          frame "HOME" {
          }
          frame "INSERT" {
          }
          frame "LBRACKET" {
          }
          frame "LCONTROL" {
          }
          frame "L ALT" {
          }
          frame "LSHIFT" {
          }
          frame "LWIN" {
          }
          frame "MINUS" {
          }
          frame "MULTIPLY" {
          }
          frame "NEXT" {
          }
          frame "NUMLOCK" {
          }
          frame "NUMPAD_0" {
          }
          frame "NUMPAD_1" {
          }
          frame "NUMPAD_2" {
          }
          frame "NUMPAD_3" {
          }
          frame "NUMPAD_4" {
          }
          frame "NUMPAD_5" {
          }
          frame "NUMPAD_6" {
          }
          frame "NUMPAD_7" {
          }
          frame "NUMPAD_8" {
          }
          frame "NUMPAD_9" {
          }
          frame "PAUSE" {
          }
          frame "PERIOD" {
          }
          frame "PRIOR (PG UP)" {
          }
          frame "RBRACKET" {
          }
          frame "RCONTROL" {
          }
          frame "RETURN" {
          }
          frame "R ALT" {
          }
          frame "RSHIFT" {
          }
          frame "RWIN" {
          }
          frame "SCROLL" {
          }
          frame "SEMICOLON" {
          }
          frame "SLASH" {
          }
          frame "SPACE" {
          }
          frame "SUBTRACT" {
          }
          frame "TAB" {
          }
          frame "DIVIDE" {
          }
          frame "DELETE" {
          }
          frame "DECIMAL" {
          }
          frame "COMMA" {
          }
          frame "CAPITAL" {
          }
          frame "BACKSLASH" {
          }
          frame "BACK" {
          }
          frame "ADD" {
          }
          frame "F15" {
          }
          frame "F14" {
          }
          frame "F13" {
          }
          frame "F12" {
          }
          frame "F11" {
          }
          frame "F10" {
          }
          frame "F9" {
          }
          frame "F8" {
          }
          frame "F7" {
          }
          frame "F6" {
          }
          frame "F5" {
          }
          frame "F4" {
          }
          frame "F3" {
          }
          frame "F2" {
          }
          frame "F1" {
          }
          frame "Z" {
          }
          frame "Y" {
          }
          frame "X" {
          }
          frame "W" {
          }
          frame "V" {
          }
          frame "U" {
          }
          frame "T" {
          }
          frame "S" {
          }
          frame "R" {
          }
          frame "Q" {
          }
          frame "P" {
          }
          frame "O" {
          }
          frame "N" {
          }
          frame "M" {
          }
          frame "L" {
          }
          frame "K" {
          }
          frame "J" {
          }
          frame "I" {
          }
          frame "H" {
          }
          frame "G" {
          }
          frame "F" {
          }
          frame "E" {
          }
          frame "D" {
          }
          frame "C" {
          }
          frame "B" {
          }
          frame "A" {
          }
          frame "9" {
          }
          frame "8" {
          }
          frame "7" {
          }
          frame "6" {
          }
          frame "5" {
          }
          frame "4" {
          }
          frame "3" {
          }
          frame "2" {
          }
          frame "1" {
          }
          frame "0" {
          }
        }
        n1134 = Bundle(w504, w503, w518, w517, 0.0) -> (w516:cluster{dbl, dbl, dbl, dbl, dbl})  [unwired: 1 in]
        n1135 = Bundle("X"=w526, "Y"=w525) -> (w520:cluster{"X":sgl, "Y":sgl})  [unwired: 1 in]
        n1136 = Divide(x=20, y=w487) -> (x/y=w490:sgl)
        n1137 = property on="Image Out" class="ImageControl"("Image Center Position"=w520) -> ()  [unwired: 2 in, 2 out]
        n1138 = call "IMAQ Convert Rectangle to ROI (Polygon)"("Rectangle"=w516) -> ("ROI Descriptor"=w514:T3)  [unwired: 7 in, 2 out]
        n1139 = Bundle("Application Font", w490, w494, w494, w494, w494, w494, TRUE, w492) -> (w496:T15)  [unwired: 1 in]
        n1140 = property on="Image Out 2" class="ImageControl"("ROI"=w514) -> ()  [unwired: 2 in, 2 out]
        n1141 = Bundle(w492, w496, w492, w492) -> (w495:T16)  [unwired: 1 in]
        n1142 = property on="Image Out" class="ImageControl"() -> ("ROI"=w469:T9)  [unwired: 2 in, 2 out]
        n1143 = Unbundle By Name(w469) -> ("Contours"=w543:T12)
        n1144 = local read "Image Out"() -> (w498:T2)
        n1145 = call "IMAQ Clear Overlay"("Image"=w498) -> ("Image Out"=w497:T2)  [unwired: 9 in, 1 out]
        n1146 = Initialize Array(0) -> (w541:i32[])  [unwired: 1 in]
        n1147 = local read "Magnification"() -> (w532:u16)
        n1148 = Array Size(array=w543) -> (size(s)=w542:i32)
        n1149 = Build Array(0.505025, 0.252522, 0.127742, 0.050345, 0.031129) -> (w533:dbl[])
        n1150 = Array Subset(array=w533, index=w532, length=1) -> (w530:dbl[])
        n1151 = property on="Image Out" class="ImageControl"() -> ("ZoomInteger"=w522:cluster{"X":i32, "Y":i32})  [unwired: 2 in, 2 out]
        n1152 = To Double Precision Float(number=w530) -> (double precision float=w529:dbl[])
        n1153 = for {
          N: w542 -> [_]
          shift-right: [w815] -> _
          shift-left: w543 -> [w815]
          shift-right: [w813] -> w528
          shift-left: w541 -> [w812]
          tunnel: w529 -> [w811]
          shift-right: [w808] -> _
          shift-left: w497 -> [w810]
          tunnel: w495 -> [w803]
          i -> [w807]
          n1154 = Index Array(array=w815, index=w807) -> (element=w824:T17)
          n1155 = Unbundle(w824) -> ("Points"=w823:i32[])  [unwired: 2 out]
          n1156 = Array To Cluster(array=w823) -> (cluster=w822:T18)
          n1157 = Unbundle(w822) -> ("Points[0]"=w802:i32, "Points[1]"=w799:i32, "Points[2]"=w814:i32, "Points[3]"=w820:i32)  [unwired: 5 out]
          n1158 = Add(x=w802, y=10) -> (x+y=w800:i32)
          n1159 = Subtract(x=w799, y=w820) -> (x-y=w819:i32)
          n1160 = Subtract(x=w802, y=w814) -> (x-y=w821:i32)
          n1161 = Square(x=w819) -> (x^2=w817:i32)
          n1162 = Square(x=w821) -> (x^2=w818:i32)
          n1163 = Add(x=w818, y=w817) -> (x+y=w816:i32)
          n1164 = Square Root(x=w816) -> (sqrt(x)=w793:dbl)
          n1165 = Multiply(x=w793, y=0.5) -> (x*y=w796:dbl)
          n1166 = Add(x=w796, y=w799) -> (x+y=w798:dbl)
          n1167 = Bundle(w800, w798) -> (w809:cluster{i32, dbl})  [unwired: 1 in]
          n1168 = Multiply(x=w793, y=w811) -> (x*y=w806:dbl[])
          n1169 = Index Array(array=w806) -> (element=w805:dbl)  [unwired: 1 in]
          n1170 = Number To Fractional String(number=w805) -> (F-format string=w804:string)  [unwired: 3 in]
          n1171 = call "IMAQ Overlay Text"("BG Color (Transparent)"=u32 0, "Text Color (black)"=u32 16448250, "Font, Size & Style"=w803, "String"=w804, "Origin"=w809, "Image"=w810) -> ("Image Out"=w808:T2)  [unwired: 4 in, 1 out]
          n1172 = Build Array (concatenate)(w812, w806) -> (w813:dbl[])
          n1173 = local write "Numeric 3"(w793) -> ()
        }
        n1174 = local write "ROI Descriptor"(w469) -> ()
        n1175 = Unbundle(w522) -> ("X"=w521:i32)  [unwired: 1 out]
        n1176 = Add Array Elements(numeric array=w528) -> (sum=w539:dbl)
        n1177 = local write "Distances"(w528) -> ()
        n1178 = local write "Total Width"(w539) -> ()
        n1179 = local write "Zoom"(w521) -> ()
        n1180 = local read "Rec: Width"() -> (w470:dbl)
        n1181 = local read "Manual"() -> (w468:bool)
        n1182 = Not(x=w468) -> (.not. x?=w466:bool)
        n1183 = local read "Total Width"() -> (w472:dbl)
        n1184 = Equal To 0?(x=w472) -> (x = 0?=w467:bool)
        n1185 = And(x=w467, y=w466) -> (x .and. y?=w465:bool)
        n1186 = case shown="True" w465 {
          tunnel: w470 -> [_ w553]
          frame False {
          }
          frame True {
            n1187 = local write "New: Width"(w553) -> ()
          }
        }
        n1188 = Or(x=w467, y=w468) -> (x .or. y?=w471:bool)
        n1189 = case shown="False" w471 {
          tunnel: w472 -> [w554 _]
          frame False {
            n1190 = local write "New: Width"(w554) -> ()
          }
          frame True {
          }
        }
      }
    }
  }
  n1191 = Build Array("DeviceID", "Fabricator", "Deposition", "Date", "Sample", "Row", "Column", "L (um)", "W (um)", "Material", "Treatment", "TC (mM)", "Solvent", "C (%)", "ST (C)", "Drops", "Wait (s)", "RT (F)", "RH (%)", "Ramp (s)", "RPM", "Accel (RPM/s)", "Time (s)", "Mobility", "On/Off", "Vt", "S.T.S") -> (→"Transformer \nHeaders":string[])
